vi "Main.vi"() -> ()   [LabVIEW 2019]
uses:
  Controls/Custom Calendar/Custom Calendar.xctl
  Controls/State Variables/Add User States.ctl
  Controls/State Variables/Edit User States.ctl
  Controls/State Variables/Add Item States.ctl
  Controls/State Variables/Edit Item States.ctl
  Controls/State Variables/Return Item States.ctl
  Controls/State Variables/Search Database States.ctl
  Controls/State Variables/User Item States.ctl
  Controls/State Variables/Main States.ctl
  Controls/State Variables/Edit Items States.ctl
  Controls/State Variables/Check Out Items States.ctl
  Controls/State Variables/Transfer Items States.ctl
  Controls/State Variables/Settings States.ctl
  Controls/State Variables/PSC Sales States.ctl
  Controls/References Cluster.ctl
  Controls/General Check Out Options.ctl
  <vilib>/event_ctls.llb/eventvkey.ctl
  <vilib>/vision/Image Controls.llb/IMAQ Image.ctl
  Controls/Table Data Types/Inventory Data Type.ctl
panel:
  in  "USER/ITEM DATA TRANSFER":T1(array[cluster])
  in  "PSC SALES MAIN STATE":T2
  in  "Settings State":T3
  in  "EMAILS SENT?":bool=TRUE
  in  "TRANSFER ITEMS STATE":T4
  in  "CHECK OUT ITEMS STATE":T5
  in  "EDIT ITEMS STATE":T6
  in  "Anticipate Graduation Year Map":map{string, i32}(c390)
  in  "Status Map":map{string, i32}(c390)
  in  "Department Map":map{string, i32}(c390)
  in  "Main State":T7
  in  "USER ITEMS STATE":T8
  in  "Search Database State":T9=enum."IDLE"
  out "Picture File Name":string
  out "BYU ID":string
  in  "RETURN ITEM STATE":T10
  in  "EDIT ITEM STATE":T11
  in  "ADD ITEM STATE":T12
  in  "EDIT USER STATE":T13
  in  "ADD USER STATE":T14
  in  "SEARCH DATABASE":bool
  in  "ADD ITEM":bool
  in  "ADD USER":bool
  in  "PSC SALES":bool
  in  "Main Pages":T15(tab)
  in  "Edit Database Settings":bool
  in  "RETURN ITEM":string
  in  "CLOSE":bool
  in  "DOWNLOAD USER PHOTO":bool
  in  "TAKE PHOTO USER":bool
  in  "User Comments":string
  in  "User Agreement":bool
  in  "CANCEL USER":bool
  in  "SAVE AND CLOSE USER":bool
  out "Add/Edit User Image":T16(plugin-control)
  out "Credit Score":string
  out "Graduation Clearance Date":string
  out "Date Added":string
  in  "Anticipated Graduation Year (Click to Select)":u16(ring) items=["2021", "2022", "2023", "2024", "2025", "2026", "2027", "2028", "2029", "2030"]
  in  "Status (Click to Select)":u16(ring) items=["Undergraduate", "Graduate", "Faculty/Staff"]
  in  "Department (Click to Select)":u16(ring) items=["ME", "EE", "CE", "CHEME", "MFGEN", "Other"]
  in  "Email (which you actually check)":string
  in  "Phone (###-###-####)":string
  in  "Last Name":string
  in  "First Name":string
  in  "BYU ID # (##-###-####)":string
  out "ADD/EDIT USER LABEL":string="ADD USER"
  in  "Camera":refnum<k21>
  in  "Reminder Notes":string
  in  "Archive Item Inputs":T17 {"Disposal Method" items=["Auction", "Sale", "Surplus", "Trash", "Other"]}
  in  "ARCHIVE ITEM":bool
  in  "CANCEL ITEM":bool
  in  "SAVE AND CLOSE ITEM":bool
  out "Most Recent Reminder Date":string
  out "Reminder Count":string
  out "Check Out Location":string
  out "Due Date":string
  out "Checked Out Date":string
  in  "Comments":string
  in  "Date Acquired":string
  in  "Serial #":string
  in  "Model #":string
  in  "Manufacturer":string
  in  "Manual":string
  in  "Location":string
  in  "Room":string
  in  "Item Description":string
  in  "BYU ICN #":string
  in  "ME #":string
  out "ADD/EDIT ITEM LABEL":string="ADD ITEM"
  in  "CANCEL RETURN ITEMS":bool
  in  "RETURN SELECTED ITEMS":bool
  in  "Item":string
  in  "What are you searching for?":u16(ring) items=["Identifier", "BYU ICN", "Item Description"]
  in  "Search Return Results":i32[](listbox)
  in  "Edit Sale Description":bool
  in  "Search Print Receipt":bool
  in  "Date Range":u16(ring) items=["Greater Than", "Less Than", "Between"]
  in  "Dates Less Than":string(xcontrol)
  in  "Dates Greater Than":string(xcontrol)
  in  "RESTORE USER":bool
  in  "CLOSE SEARCH":bool
  in  "EXPORT TO CLIPBOARD":bool
  in  "OPEN ITEM":bool
  in  "Sales Tracking Column Selector":T18={"SALE ID #"=TRUE, "BYU ID CARD #"=TRUE, "Sale Description"=TRUE, "Grand Total"=TRUE, "SALE DATE"=TRUE, "ITEM DESCRIPTION"=TRUE, "ITEM UNIT PRICE"=TRUE, "ITEM TOTAL PRICE"=TRUE, "ITEM QUANTITY"=TRUE, "SALE SEMESTER"=TRUE}
  in  "User Archive Column Selector":T19={"BYU ID #"=TRUE, "FIRST NAME"=TRUE, "LAST NAME"=TRUE, "PHONE NUMBER"=FALSE, "EMAIL"=FALSE, "DEPARTMENT"=TRUE, "STATUS"=TRUE, "ANTICIPATED GRADUATION YEAR"=TRUE, "CREDIT SCORE"=FALSE, "DATE ADDED"=TRUE, "GRADUATION CLEARANCE DATE"=TRUE, "USER PROFILE PICTURE PATH"=FALSE, "DATE ARCHIVED"=TRUE}
  in  "Inventory Archive Column Selector":T20={"DATE DISPOSED"=TRUE, "DISPOSAL METHOD"=TRUE, "AUCTION #"=TRUE, "DATE INVENTORY OFFICE EMAILED"=TRUE, "DISPOSAL NOTES"=TRUE, "IDENTIFIER"=TRUE, "BYU ICN #"=TRUE, "ITEM"=TRUE, "COMMENTS"=TRUE, "BUILDING/ROOM"=FALSE, "LOCATION IN ROOM"=FALSE, "MANUAL"=FALSE, "MANUFACTURER"=FALSE, "MODEL #"=FALSE, "SERIAL #"=FALSE, "DATE ACQUIRED"=TRUE}
  in  "User Column Selector":T21={"BYU ID #"=TRUE, "FIRST NAME"=TRUE, "LAST NAME"=TRUE, "PHONE NUMBER"=TRUE, "EMAIL"=TRUE, "DEPARTMENT"=TRUE, "GRADUATION STATUS"=TRUE, "ANTICIPATED GRADUATION YEAR"=FALSE, "CREDIT SCORE"=TRUE, "DATE ADDED"=FALSE, "GRADUATION CLEARANCE DATE"=FALSE, "PICTURE FILE NAME"=FALSE, "PICTURE FILE NAME 2"=FALSE}
  in  "Inventory Column Selector":T22={"IDENTIFIER"=TRUE, "BYU ICN #"=TRUE, "ITEM"=TRUE, "BUILDING/ROOM"=FALSE, "LOCATION IN ROOM"=FALSE, "MANUAL"=TRUE, "MANUFACTURER"=FALSE, "MODEL #"=FALSE, "SERIAL #"=FALSE, "DATE ACQUIRED"=FALSE, "BYU ID"=TRUE, "FIRST NAME"=TRUE, "LAST NAME"=TRUE, "CHECK OUT LOCATION"=TRUE, "CHECKED OUT DATE"=TRUE, "DUE DATE"=TRUE, "REMINDER COUNT"=TRUE, "MOST RECENT REMINDER DATE"=TRUE, "COMMENTS"=FALSE, "REMINDER NOTES"=FALSE}
  in  "COLUMNS TO VIEW":bool
  in  "OPEN USER":bool
  in  "Search Database Results":i32(listbox)
  in  "Column to Sort By":u16(ring) items=["BYU ID #", "First Name", "Last Name", "Phone Number", "Email", "Department", "Graduation Status", "Anticipated Graduation Year", "Credit Score", "Date Added", "Graduation Clearance Date", "User Profile Picture Path"]
  in  "Column to Search In":u16(ring) items=["BYU ID #", "First Name", "Last Name", "Phone Number", "Email", "Department", "Graduation Status", "Anticipated Graduation Year", "Credit Score", "Date Added", "Graduation Clearance Date", "User Profile Picture Path"]
  in  "What to Search For:":string
  in  "Where to Search":u16(ring) items=["Inventory", "Users", "Checked Out Items", "Inventory Archive", "User Archive", "Checked In Archive", "Sales Tracking", "Sales Archive"]
  in  "Checked In Archive Selector":T23={"ME #/ID #"=TRUE, "BYU ICN #"=TRUE, "ITEM DESCRIPTION"=TRUE, "BUILDING/ROOM"=FALSE, "LOCATION IN ROOM"=FALSE, "MANUAL"=TRUE, "MANUFACTURER"=FALSE, "MODEL #"=FALSE, "SERIAL #"=FALSE, "DATE ACQUIRED"=FALSE, "BYU ID #"=TRUE, "FIRST NAME"=TRUE, "LAST NAME"=TRUE, "CHECK OUT LOCATION"=TRUE, "CHECKED OUT DATE"=TRUE, "DUE DATE"=TRUE, "DATE RETURNED"=TRUE, "REMINDER COUNT"=FALSE, "MOST RECENT REMINDER DATE"=FALSE, "COMMENTS"=FALSE, "REMINDER NOTES"=FALSE}
  in  "SEE USER INFO COMMENTS":bool
  in  "User Info Comments":string
  in  "CHECK OUT ITEMS":bool
  in  "LOG OUT USER":bool
  in  "ARCHIVE USER":bool
  in  "EDIT USER":bool
  in  "EDIT SELECTED ITEMS":bool
  in  "TRANSFER SELECTED ITEMS":bool
  in  "USER RETURN SELECTED ITEMS":bool
  in  "User's Checked Out Items":i32[](listbox)
  in  "USER'S INFO":T24
  in  "USER EXPORT TO CLIPBOARD":bool
  in  "Altered Item Description":string
  in  "Possible Items":i32(listbox)
  in  "FINISH CHECK OUT ITEMS":bool
  in  "REMOVE SELECTED ITEMS":bool
  in  "CANCEL CHECK OUT ITEMS":bool
  in  "Items to be Checked Out":i32[](listbox)
  in  "Enter Item:":string
  in  "Check Out Location Selection":string
  in  "CHECK OUT STATICS":bool
  in  "CHECK OUT TODAY":bool
  in  "CHECK OUT END OF SEMESTER":bool
  in  "CHECK OUT MEASUREMENTS":bool
  in  "CHECK OUT MECHATRONICS":bool
  in  "Check Out Items Due Date":string(xcontrol)
  in  "New Item Description":string
  in  "New Reminder Notes":string
  in  "EDIT ITEMS SAVE AND CLOSE":bool
  in  "Items to Edit":i32[](listbox)
  in  "CANCEL EDIT ITEMS":bool
  in  "EDIT ITEMS REMOVE SELECTED ITEMS":bool
  in  "New Check Out Location":string
  in  "Edit Items Due Date":string(xcontrol)
  in  "EDIT ITEMS END OF SEMESTER":bool
  in  "EDIT ITEMS MECHATRONICS":bool
  in  "EDIT ITEMS STATICS":bool
  in  "EDIT ITEMS MEASUREMENTS":bool
  in  "TODAY EDIT ITEMS":bool
  in  "TRANSFER ITEMS":bool
  in  "Matching Individuals":i32(listbox)
  in  "TRANSFER ITEM REMOVE SELECTED ITEMS":bool
  in  "CANCEL TRANSFER ITEMS":bool
  in  "Items to be Transferred":i32[](listbox)
  in  "What to Match":u16(ring) items=["Last Name", "First Name", "BYU ID #"]
  in  "Search Parameter":string
  in  "Print Receipt":bool
  in  "CUSTOM ITEM":bool
  in  "Item List":i32[](listbox)
  in  "SAVE SALE AND CLOSE":bool
  out "Grand Total":string
  in  "BYU ID CARD #":string
  in  "Sale Description":string
  in  "Items to be Sold":i32[](listbox)
  in  "CANCEL ITEM SALE":bool
  in  "REMOVE SELECTED ITEMS SALES":bool
  in  "RUN CHARGE":bool
  in  "Scan or Enter Item Name":string
  in  "REMOVE SALE ITEM":bool
  in  "ADD NEW SALES ITEM":bool
  in  "PSC Sales Item Spreadsheet":string[][](table)
  in  "CANCEL EDIT SETTINGS":bool
  in  "Update Settings":bool
  in  "PSC Database Settings":string[][](table)
  in  "Enable or Disable Emails \n(Make sure only one computer has this enabled)":enum16{"ENABLE EMAILS", "DISABLE EMAILS"}(ring)
  # "Project Support Center\nDatabase Version 5.1.11"
  # "By checking this box I agree to return items in a prompt manner \nand will pay any late fees or replacement costs for late, broken or non-returned items.\nI also acknowledge that failure to return items could inhibit my ability to register for \nclasses and graduate - 12/5/2023"
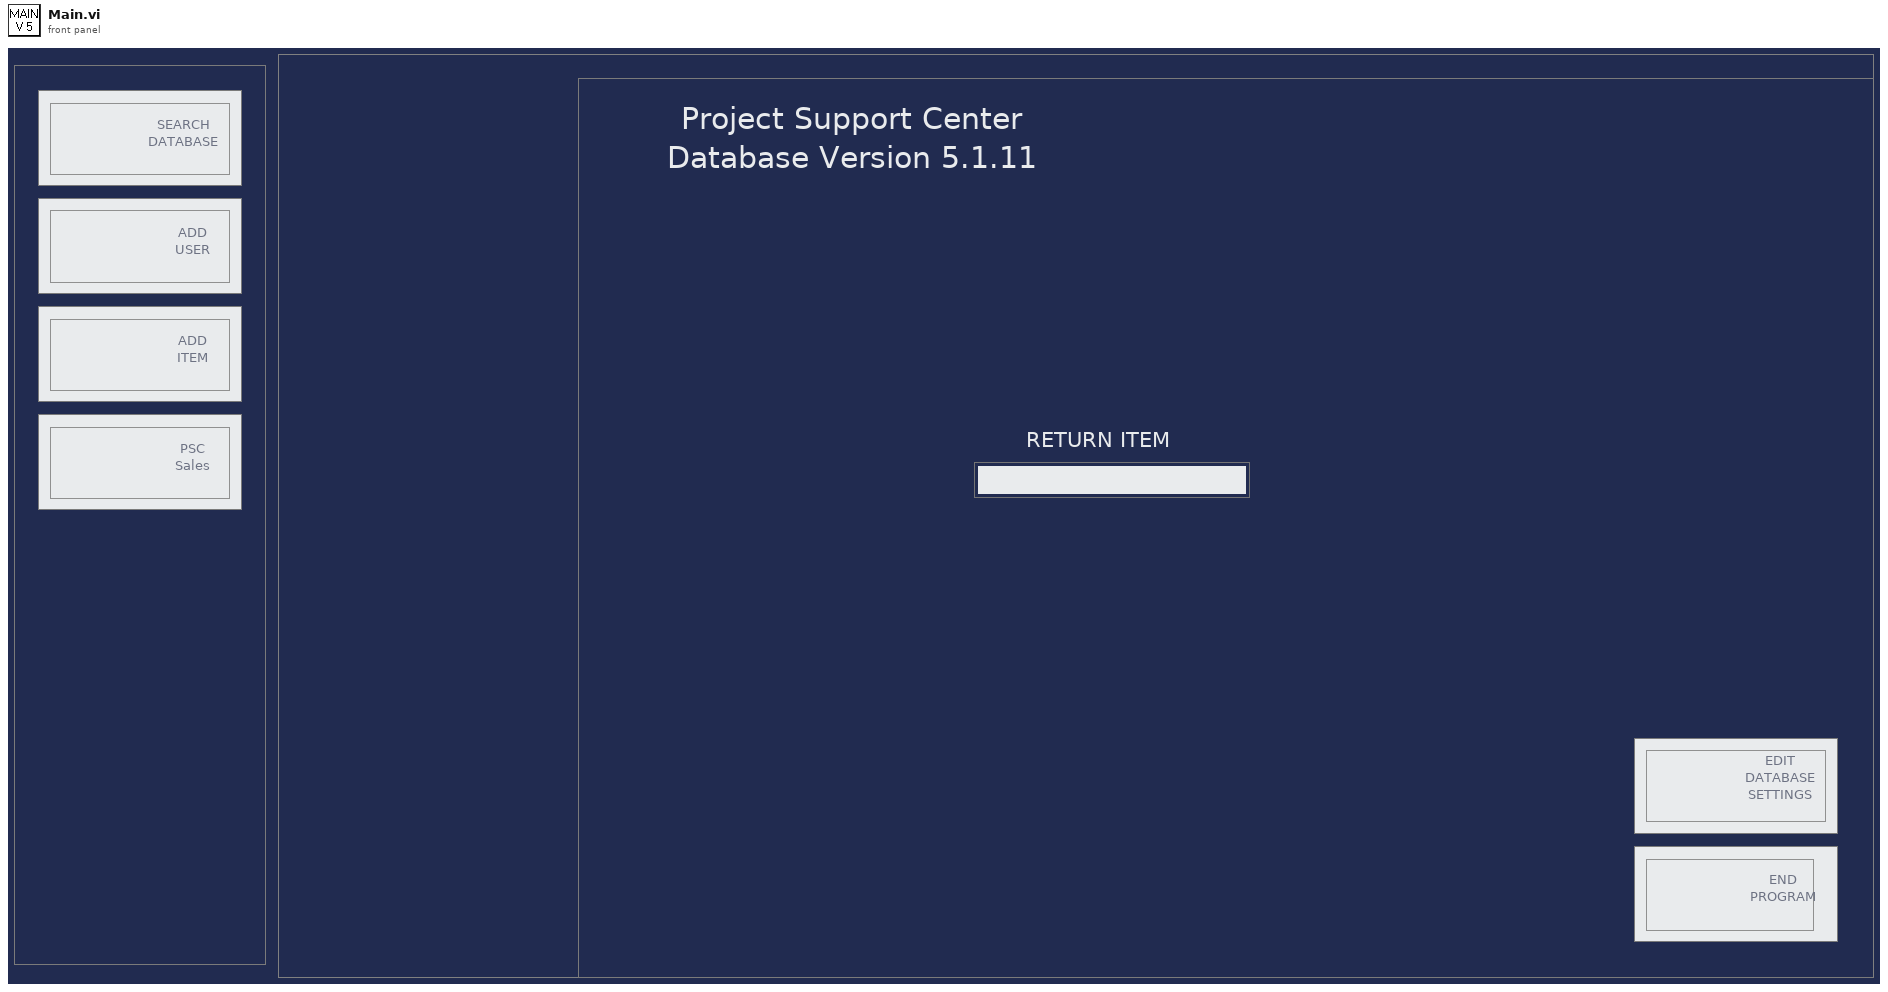
[diagram p1: front panel]
types:
  T1 = cluster{"DATA TYPE":enum16{"BYU ID", "ME#/IDENTIFIER", "BYU ICN"}, "DATA":string}[]
  T2 = typedef "PSC Sales States.ctl" = enum16{"INIT", "IDLE", "SEARCH ITEM LIST", "CUSTOM ITEM", "GET QUANTITY", "REMOVE ITEMS", "RUN CHARGE", "PRINT RECEIPT", "SAVE SALE", "END"}
  T3 = typedef "Settings States.ctl" = enum16{"INIT", "IDLE", "ADD SALE ITEM", "REMOVE SALE ITEM", "UPDATE SETTINGS", "END"}
  T4 = typedef "Transfer Items States.ctl" = enum16{"INIT", "IDLE", "FIND USER", "CONFIRM SELECTION", "REMOVE ITEMS", "TRANSFER ITEMS", "END"}
  T5 = typedef "Check Out Items States.ctl" = enum16{"INIT", "IDLE", "UPDATE SEARCH", "ADD ITEM", "EDIT DUE DATE", "EDIT LOCATION", "REMOVE ITEMS", "EDIT ITEM DESCRIPTION", "CHECK OUT ITEMS", "END"}
  T6 = typedef "Edit Items States.ctl" = enum16{"INIT", "IDLE", "EDIT DUE DATE", "EDIT LOCATION", "EDIT NOTES", "EDIT ITEM DESCRIPTION", "REMOVE ITEMS", "EDIT ITEMS", "END"}
  T7 = typedef "Main States.ctl" = enum16{"INIT", "IDLE", "ADD USER", "EDIT USER", "ADD ITEM", "EDIT ITEM", "RETURN ITEMS", "SEARCH DATABASE", "USER ITEMS", "EDIT ITEMS", "CHECK OUT ITEMS", "TRANSFER ITEMS", "PSC SALES", "ATRIUM", "INVENTORY TRACKING", "SETTINGS", "REMINDER EMAILS", "END"}
  T8 = typedef "User Item States.ctl" = enum16{"INIT", "IDLE", "GET USER ITEMS", "EDIT SELECTED ITEMS", "RETURN SELECTED ITEMS", "TRANSFER SELECTED ITEMS", "EDIT ALL ITEMS", "RETURN ALL ITEMS", "TRANSFER ALL ITEMS", "CHECK OUT ITEMS", "EDIT USER", "ARCHIVE USER", "END"}
  T9 = typedef "Search Database States.ctl" = enum16{"INIT", "IDLE", "UPDATE COLUMNS", "SEARCH DATABASE", "OPEN USER", "OPEN ITEM", "RESTORE USER", "PRINT SALE RECEIPT", "EDIT SALE DESCRIPTION", "END"}
  T10 = typedef "Return Item States.ctl" = enum16{"INIT", "IDLE", "SEARCH ITEMS", "RETURN ITEMS", "END"}
  T11 = typedef "Edit Item States.ctl" = enum16{"INIT", "IDLE", "EDIT ITEM", "ARCHIVE ITEM", "END"}
  T12 = typedef "Add Item States.ctl" = enum16{"INIT", "IDLE", "ADD ITEM", "END"}
  T13 = typedef "Edit User States.ctl" = enum16{"INIT", "IDLE", "TAKE PHOTO", "GET PHOTO", "EDIT USER", "END"}
  T14 = typedef "Add User States.ctl" = enum16{"INIT", "IDLE", "TAKE PHOTO", "GET PHOTO", "ADD USER", "END"}
  T15 = enum32{"IDLE", "ADD/EDIT USER", "ADD/EDIT ITEM", "RETURN ITEMS", "SEARCH DATABASE", "USER ITEMS", "CHECK OUT ITEMS", "EDIT ITEMS", "TRANSFER ITEMS", "PSC SALES", "ATRIUM", "INVENTORY TRACKING", "SETTINGS"}
  T16 = typedef "IMAQ Image.ctl" = refnum<image>
  T17 = cluster{"Disposal Date":string, "Disposal Method":u16, "Auction # / Other":string, "Date Disposal Email Sent":string, "Disposal Notes":string}
  T18 = cluster{"SALE ID #":bool, "BYU ID CARD #":bool, "Sale Description":bool, "Grand Total":bool, "SALE DATE":bool, "ITEM DESCRIPTION":bool, "ITEM UNIT PRICE":bool, "ITEM TOTAL PRICE":bool, "ITEM QUANTITY":bool, "SALE SEMESTER":bool}
  T19 = cluster{"BYU ID #":bool, "FIRST NAME":bool, "LAST NAME":bool, "PHONE NUMBER":bool, "EMAIL":bool, "DEPARTMENT":bool, "STATUS":bool, "ANTICIPATED GRADUATION YEAR":bool, "CREDIT SCORE":bool, "DATE ADDED":bool, "GRADUATION CLEARANCE DATE":bool, "USER PROFILE PICTURE PATH":bool, "DATE ARCHIVED":bool}
  T20 = cluster{"DATE DISPOSED":bool, "DISPOSAL METHOD":bool, "AUCTION #":bool, "DATE INVENTORY OFFICE EMAILED":bool, "DISPOSAL NOTES":bool, "IDENTIFIER":bool, "BYU ICN #":bool, "ITEM":bool, "COMMENTS":bool, "BUILDING/ROOM":bool, "LOCATION IN ROOM":bool, "MANUAL":bool, "MANUFACTURER":bool, "MODEL #":bool, "SERIAL #":bool, "DATE ACQUIRED":bool}
  T21 = cluster{"BYU ID #":bool, "FIRST NAME":bool, "LAST NAME":bool, "PHONE NUMBER":bool, "EMAIL":bool, "DEPARTMENT":bool, "GRADUATION STATUS":bool, "ANTICIPATED GRADUATION YEAR":bool, "CREDIT SCORE":bool, "DATE ADDED":bool, "GRADUATION CLEARANCE DATE":bool, "PICTURE FILE NAME":bool, "PICTURE FILE NAME 2":bool}
  T22 = cluster{"IDENTIFIER":bool, "BYU ICN #":bool, "ITEM":bool, "BUILDING/ROOM":bool, "LOCATION IN ROOM":bool, "MANUAL":bool, "MANUFACTURER":bool, "MODEL #":bool, "SERIAL #":bool, "DATE ACQUIRED":bool, "BYU ID":bool, "FIRST NAME":bool, "LAST NAME":bool, "CHECK OUT LOCATION":bool, "CHECKED OUT DATE":bool, "DUE DATE":bool, "REMINDER COUNT":bool, "MOST RECENT REMINDER DATE":bool, "COMMENTS":bool, "REMINDER NOTES":bool}
  T23 = cluster{"ME #/ID #":bool, "BYU ICN #":bool, "ITEM DESCRIPTION":bool, "BUILDING/ROOM":bool, "LOCATION IN ROOM":bool, "MANUAL":bool, "MANUFACTURER":bool, "MODEL #":bool, "SERIAL #":bool, "DATE ACQUIRED":bool, "BYU ID #":bool, "FIRST NAME":bool, "LAST NAME":bool, "CHECK OUT LOCATION":bool, "CHECKED OUT DATE":bool, "DUE DATE":bool, "DATE RETURNED":bool, "REMINDER COUNT":bool, "MOST RECENT REMINDER DATE":bool, "COMMENTS":bool, "REMINDER NOTES":bool}
  T24 = cluster{"BYU ID #":string, "First Name":string, "Last Name":string, "Phone Number":string, "Email":string, "Department":string, "Graduation Status":string, "Grad Year":string, "Credit Score":string, "Date Added":string, "Graduation Clearance Date":string, "User Items Photo":T16}
  T25 = typedef "References Cluster.ctl" = cluster{"MAIN PAGES":refnum<vi>, "ADD/EDIT ITEM REFERENCES":cluster{"Identifier":refnum<vi>, "BYU ICN #":refnum<vi>, "Item Description":refnum<vi>, "Comments":refnum<vi>, "Checked Out Date":refnum<vi>, "Due Date":refnum<vi>, "Check Out Location":refnum<vi>, "Reminder Count":refnum<vi>, "Most Recent Reminder Date":refnum<vi>, "BYU ID #":refnum<vi>, "Building/Room":refnum<vi>, "Location in Room":refnum<vi>, "Manual":refnum<vi>, "Manufacturer":refnum<vi>, "Model #":refnum<vi>, "Serial #":refnum<vi>, "Date Acquired":refnum<vi>, "ADD/EDIT ITEM LABEL":refnum<vi>, "ARCHIVE ITEM":refnum<vi>, "Archive Item Inputs":refnum<vi>, "Reminder Notes":refnum<vi>}, "ADD/EDIT USER REFERENCES":cluster{"BYU ID # (##-###-####)":refnum<vi>, "First Name":refnum<vi>, "Last Name":refnum<vi>, "Phone Number (###-###-####)":refnum<vi>, "Email":refnum<vi>, "Department":refnum<vi>, "Graduation Status":refnum<vi>, "Anticipated Graduation Year":refnum<vi>, "Credit Score":refnum<vi>, "Date Added":refnum<vi>, "Graduation Clearance Date":refnum<vi>, "Picture File Name":refnum<vi>, "ADD/EDIT USER LABEL":refnum<vi>, "Department Map":refnum<vi>, "Status Map":refnum<vi>, "Anticipated Graduation Year Map":refnum<vi>, "User Agreement":refnum<vi>, "User Comments":refnum<vi>, "Camera":refnum<vi>}, "RETURN ITEM REFERENCES":cluster{"Item or Person:":refnum<vi>, "Search Return Results":refnum<vi>, "What are you searching for?":refnum<vi>}, "SEARCH DATABASE REFERENCES":cluster{"What to Search For:":refnum<vi>, "Where to Search":refnum<vi>, "Column to Search In":refnum<vi>, "Column to Sort By":refnum<vi>, "Search Database Results":refnum<vi>, "Inventory Column Selector":refnum<vi>, "User Column Selector":refnum<vi>, "Inventory Archive Column Selector":refnum<vi>, "User Archive Column Selector":refnum<vi>, "Sales Tracking Column Selector":refnum<vi>, "Checked In Archive Column Selector":refnum<vi>, "Restore User":refnum<vi>, "Date Range":refnum<vi>, "Dates Less Than":refnum<vi>, "Dates Greater Than":refnum<vi>, "Search Print Receipt":refnum<vi>, "Edit Sale Description":refnum<vi>}, "USER ITEMS REFERENCES":cluster{"USER'S INFORMATION":refnum<vi>, "User's Checked Out Items":refnum<vi>, "User Info Comments":refnum<vi>, "SEE USER INFO COMMENTS":refnum<vi>}, "EDIT ITEMS REFERENCES":cluster{"New Check Out Location":refnum<vi>, "Items to Edit":refnum<vi>, "Edit Items Due Date":refnum<vi>, "New Reminder Notes":refnum<vi>, "New Item Description":refnum<vi>}, "CHECK OUT ITEMS REFERENCES":cluster{"Enter Item:":refnum<vi>, "Check Out Items Due Date":refnum<vi>, "Check Out Location":refnum<vi>, "Items to be Checked Out":refnum<vi>, "Possible Items":refnum<vi>, "Altered Item Description":refnum<vi>}, "TRANSFER ITEMS REFERENCES":cluster{"Search Parameter":refnum<vi>, "What to Match":refnum<vi>, "Matching Individuals":refnum<vi>, "Items to be Transferred":refnum<vi>}, "SETTINGS REFERENCES":cluster{"PSC Database Settings":refnum<vi>, "PSC Sales Item Spreadsheet":refnum<vi>}, "PSC SALES REFERENCES":cluster{"BYU ID CARD #":refnum<vi>, "Sale Description":refnum<vi>, "Scan or Enter Item Name":refnum<vi>, "Items to be Sold":refnum<vi>, "Grand Total":refnum<vi>, "Item List":refnum<vi>}}
  T26 = cluster{"Identifier":refnum<vi>, "BYU ICN #":refnum<vi>, "Item Description":refnum<vi>, "Comments":refnum<vi>, "Checked Out Date":refnum<vi>, "Due Date":refnum<vi>, "Check Out Location":refnum<vi>, "Reminder Count":refnum<vi>, "Most Recent Reminder Date":refnum<vi>, "BYU ID #":refnum<vi>, "Building/Room":refnum<vi>, "Location in Room":refnum<vi>, "Manual":refnum<vi>, "Manufacturer":refnum<vi>, "Model #":refnum<vi>, "Serial #":refnum<vi>, "Date Acquired":refnum<vi>, "ADD/EDIT ITEM LABEL":refnum<vi>, "ARCHIVE ITEM":refnum<vi>, "Archive Item Inputs":refnum<vi>, "Reminder Notes":refnum<vi>}
  T27 = cluster{"BYU ID # (##-###-####)":refnum<vi>, "First Name":refnum<vi>, "Last Name":refnum<vi>, "Phone Number (###-###-####)":refnum<vi>, "Email":refnum<vi>, "Department":refnum<vi>, "Graduation Status":refnum<vi>, "Anticipated Graduation Year":refnum<vi>, "Credit Score":refnum<vi>, "Date Added":refnum<vi>, "Graduation Clearance Date":refnum<vi>, "Picture File Name":refnum<vi>, "ADD/EDIT USER LABEL":refnum<vi>, "Department Map":refnum<vi>, "Status Map":refnum<vi>, "Anticipated Graduation Year Map":refnum<vi>, "User Agreement":refnum<vi>, "User Comments":refnum<vi>, "Camera":refnum<vi>}
  T28 = cluster{"Item or Person:":refnum<vi>, "Search Return Results":refnum<vi>, "What are you searching for?":refnum<vi>}
  T29 = cluster{"What to Search For:":refnum<vi>, "Where to Search":refnum<vi>, "Column to Search In":refnum<vi>, "Column to Sort By":refnum<vi>, "Search Database Results":refnum<vi>, "Inventory Column Selector":refnum<vi>, "User Column Selector":refnum<vi>, "Inventory Archive Column Selector":refnum<vi>, "User Archive Column Selector":refnum<vi>, "Sales Tracking Column Selector":refnum<vi>, "Check In Archive Column Selector":refnum<vi>, "Restore User":refnum<vi>, "Date Range":refnum<vi>, "Dates Less Than":refnum<vi>, "Dates Greater Than":refnum<vi>, "Search Print Receipt":refnum<vi>, "Edit Sale Description":refnum<vi>}
  T30 = cluster{"USER'S INFORMATION":refnum<vi>, "User's Checked Out Items":refnum<vi>, "User Info Comments":refnum<vi>, "SEE USER INFO COMMENTS":refnum<vi>}
  T31 = cluster{"New Check Out Location":refnum<vi>, "Items to Edit":refnum<vi>, "Edit Items Due Date":refnum<vi>, "New Reminder Notes":refnum<vi>, "New Item Description":refnum<vi>}
  T32 = cluster{"Enter Item:":refnum<vi>, "Check Out Items Due Date":refnum<vi>, "Check Out Location":refnum<vi>, "Items to be Checked Out":refnum<vi>, "Possible Items":refnum<vi>, "Altered Item Description":refnum<vi>}
  T33 = cluster{"Search Parameter":refnum<vi>, "What to Match":refnum<vi>, "Matching Individuals":refnum<vi>, "Items to be Transferred":refnum<vi>}
  T34 = cluster{"PSC Database Settings":refnum<vi>, "PSC Sales Spreadsheet":refnum<vi>}
  T35 = cluster{"BYU ID CARD #":refnum<vi>, "Sale Description":refnum<vi>, "Scan Barcode":refnum<vi>, "Items to be Sold":refnum<vi>, "Grand Total":refnum<vi>, "Item List":refnum<vi>}
  T36 = cluster{"BYU ID #":string, "First Name":string, "Last Name":string, "Phone Number":string, "Email":string, "Department":u16, "Graduation Status":u16, "Anticipated Graduation Year":u16, "Credit Score":string, "Date Added":string, "Graduation Clearance Date":string, "Picture File Name":string, "User Comments":string}
  T37 = cluster{"Identifier":string, "BYU ICN #":string, "Item Description":string, "Comments":string, "Checked Out Date":string, "Due Date":string, "Check Out Location":string, "Reminder Count":string, "Most Recent Reminder Date":string, "BYU ID #":string, "Building/Room":string, "Location in Room":string, "Manual":string, "Manufacturer":string, "Model #":string, "Serial #":string, "Date Acquired":string, "Reminder Notes":string}
  T38 = typedef "Inventory Data Type.ctl" = cluster{"Identifier":string, "BYU ICN #":string, "Item Description":string, "Comments":string, "Checked Out Date":string, "Due Date":string, "Check Out Location":string, "Reminder Count":i32, "Most Recent Reminder Date":string, "BYU ID #":string, "Building/Room":string, "Location in Room":string, "Manual":string, "Manufacturer":string, "Model #":string, "Serial #":string, "Date Acquired":string, "Reminder Notes":string}
  T39 = cluster{"DATA TYPE":enum16{"BYU ID", "ME#/IDENTIFIER", "BYU ICN"}, "DATA":string}
  T40 = enum8{"Enabled", "Disabled", "Disabled and Grayed Out"}
  T41 = typedef "General Check Out Options.ctl" = enum16{"TODAY", "END OF SEMESTER", "MEASUREMENTS", "MECHATRONICS", "STATICS"}
  T42 = typedef "eventvkey.ctl" = enum16{"ASCII", "Enter", "Return", "Shift", "Ctrl", "Alt", "Cmd", "Opt", "Caps", "NumLock", "Clear", "Break", "Up", "Down", "Left", "Right", "Insert", "Delete", "Home", "End", "PageUp", "PageDown", "Escape", "Help", "Pause", "ScrollLock", "F1", "F2", "F3", "F4", "F5", "F6", "F7", "F8", "F9", "F10", "F11", "F12", "F13", "F14", "F15", "F16", "F17", "F18", "F19", "F20", "F21", "F22", "F23", "F24", "Play", "VolumeUp", "VolumeDown", "Mute", "Two Byte Char"}
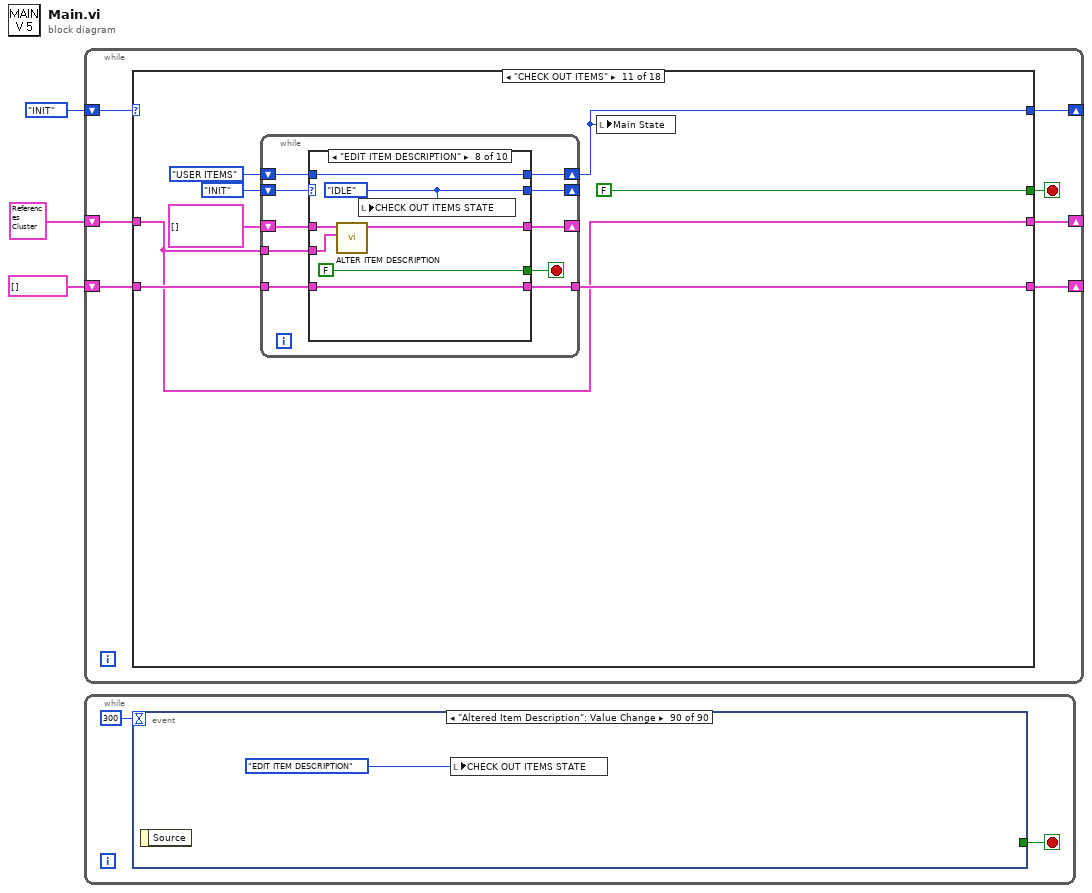
[diagram p0: block diagram]
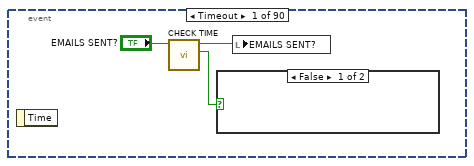
[diagram p2: hidden frame]
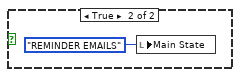
[diagram p3: hidden frame]
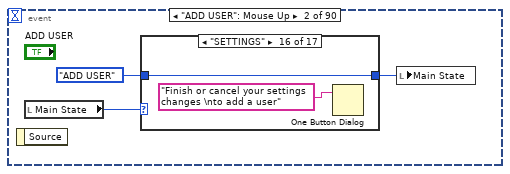
[diagram p4: hidden frame]
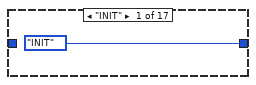
[diagram p5: hidden frame]
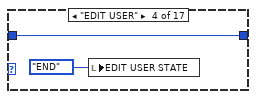
[diagram p8: hidden frame]
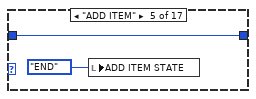
[diagram p9: hidden frame]
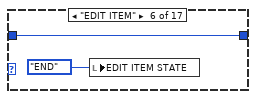
[diagram p10: hidden frame]
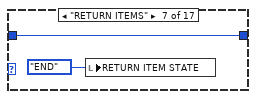
[diagram p11: hidden frame]
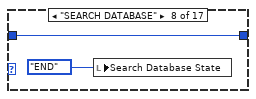
[diagram p12: hidden frame]
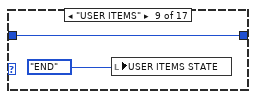
[diagram p13: hidden frame]
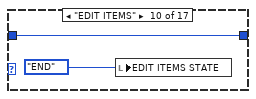
[diagram p14: hidden frame]
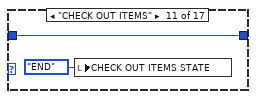
[diagram p15: hidden frame]
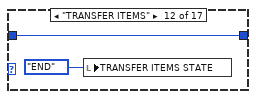
[diagram p16: hidden frame]
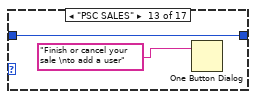
[diagram p17: hidden frame]
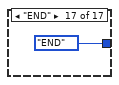
[diagram p20: hidden frame]
diagram:
  n1 = while {
    shift-right: [w6] -> _
    shift-left: Main_States."INIT" -> [w4]
    shift-right: [w8] -> _
    shift-left: T25 {"MAIN PAGES"=refnum, "ADD/EDIT ITEM REFERENCES"={"Identifier"=refnum, "BYU ICN #"=refnum, "Item Description"=refnum, "Comments"=refnum, "Checked Out Date"=refnum, "Due Date"=refnum, "Check Out Location"=refnum, "Reminder Count"=refnum, "Most Recent Reminder Date"=refnum, "BYU ID #"=refnum, "Building/Room"=refnum, "Location in Room"=refnum, "Manual"=refnum, "Manufacturer"=refnum, "Model #"=refnum, "Serial #"=refnum, "Date Acquired"=refnum, "ADD/EDIT ITEM LABEL"=refnum, "ARCHIVE ITEM"=refnum, "Archive Item Inputs"=refnum, "Reminder Notes"=refnum}, "ADD/EDIT USER REFERENCES"={"BYU ID # (##-###-####)"=refnum, "First Name"=refnum, "Last Name"=refnum, "Phone Number (###-###-####)"=refnum, "Email"=refnum, "Department"=refnum, "Graduation Status"=refnum, "Anticipated Graduation Year"=refnum, "Credit Score"=refnum, "Date Added"=refnum, "Graduation Clearance Date"=refnum, "Picture File Name"=refnum, "ADD/EDIT USER LABEL"=refnum, "Department Map"=refnum, "Status Map"=refnum, "Anticipated Graduation Year Map"=refnum, "User Agreement"=refnum, "User Comments"=refnum, "Camera"=refnum}, "RETURN ITEM REFERENCES"={"Item or Person:"=refnum, "Search Return Results"=refnum, "What are you searching for?"=refnum}, "SEARCH DATABASE REFERENCES"={"What to Search For:"=refnum, "Where to Search"=refnum, "Column to Search In"=refnum, "Column to Sort By"=refnum, "Search Database Results"=refnum, "Inventory Column Selector"=refnum, "User Column Selector"=refnum, "Inventory Archive Column Selector"=refnum, "User Archive Column Selector"=refnum, "Sales Tracking Column Selector"=refnum, "Checked In Archive Column Selector"=refnum, "Restore User"=refnum, "Date Range"=refnum, "Dates Less Than"=refnum, "Dates Greater Than"=refnum, "Search Print Receipt"=refnum, "Edit Sale Description"=refnum}, "USER ITEMS REFERENCES"={"USER'S INFORMATION"=refnum, "User's Checked Out Items"=refnum, "User Info Comments"=refnum, "SEE USER INFO COMMENTS"=refnum}, "EDIT ITEMS REFERENCES"={"New Check Out Location"=refnum, "Items to Edit"=refnum, "Edit Items Due Date"=refnum, "New Reminder Notes"=refnum, "New Item Description"=refnum}, "CHECK OUT ITEMS REFERENCES"={"Enter Item:"=refnum, "Check Out Items Due Date"=refnum, "Check Out Location"=refnum, "Items to be Checked Out"=refnum, "Possible Items"=refnum, "Altered Item Description"=refnum}, "TRANSFER ITEMS REFERENCES"={"Search Parameter"=refnum, "What to Match"=refnum, "Matching Individuals"=refnum, "Items to be Transferred"=refnum}, "SETTINGS REFERENCES"={"PSC Database Settings"=refnum, "PSC Sales Item Spreadsheet"=refnum}, "PSC SALES REFERENCES"={"BYU ID CARD #"=refnum, "Sale Description"=refnum, "Scan or Enter Item Name"=refnum, "Items to be Sold"=refnum, "Grand Total"=refnum, "Item List"=refnum}} ("REFERENCES") -> [w9]
    shift-right: [w5] -> _
    shift-left: T1 [] ("USER/ITEM DATA TRANSFER") -> [w7]
    stop <- w10 stop-if-true
    n2 = case shown="\"CHECK OUT ITEMS\"" w4 {
      tunnel: [FALSE FALSE FALSE FALSE FALSE FALSE w420 FALSE FALSE FALSE FALSE FALSE FALSE FALSE FALSE FALSE FALSE TRUE] -> w10
      tunnel: w9 -> [w15 w166 w174 w263 w338 w376 w421 w450 w543 w658 w743 w840 w922 w965 w970 w976 w1014 w1018]
      tunnel: [w14 w166 w174 w263 w338 w376 w421 w450 w543 w658 w743 w840 w922 w965 w970 w973 w1014 w1018] -> w8
      tunnel: w7 -> [w12 _ w169 w261 w334 w374 w419 w452 w541 w652 w747 w843 w923 w964 w969 w975 w1015 _]
      tunnel: [w11 "Main State" w171 w258 w335 w372 w418 w446 w539 w654 w742 w836 w919 w963 w967 w971 w1012 Main_States."END"] -> w6
      tunnel: [w12 "USER/ITEM DATA TRANSFER" w168 w257 w334 w374 w419 w449 w538 w656 w745 w841 w923 w964 w969 w974 w1015 T1 [] ("USER/ITEM DATA TRANSFER")] -> w5
      frame "INIT", Default {
        w11 = Main_States."IDLE"
        n3 = for {
          N: 12 -> [_]
          shift-right: [w17] -> w14
          shift-left: w15 -> [w18]
          i -> [w19]
          n4 = case shown="7" w19 {
            tunnel: w18 -> [w27 w52 w62 w78 w103 w111 w119 w124 w132 w145 w151 w157]
            tunnel: [w25 w50 w68 w76 w91 w106 w117 w125 w133 w145 w150 w154] -> w17
            frame 0, Default {
              n5 = control-ref of="RETURN ITEM"() -> (w22:refnum<vi>)
              n6 = control-ref of="USER/ITEM DATA TRANSFER"() -> (w23:refnum<vi>)
              n7 = property class="Str"(reference=w22, "Value"="") -> ()  [unwired: 1 in, 2 out]
              n8 = local write "Main State"(Main_States."IDLE") -> ()
              n9 = property class="Arr (strict)"(reference=w23, "Value"=T1 []) -> ()  [unwired: 1 in, 2 out]
              n10 = control-ref of="Main Pages"() -> (w26:refnum<vi>)
              n11 = Bundle By Name(cluster=w27, "MAIN PAGES"=w26) -> (w25:T25)
            }
            frame 1 {
              n12 = control-ref of="ME #"() -> (w49:refnum<vi>)
              n13 = control-ref of="BYU ICN #"() -> (w48:refnum<vi>)
              n14 = control-ref of="Item Description"() -> (w47:refnum<vi>)
              n15 = control-ref of="Comments"() -> (w46:refnum<vi>)
              n16 = control-ref of="Checked Out Date"() -> (w45:refnum<vi>)
              n17 = control-ref of="Due Date"() -> (w44:refnum<vi>)
              n18 = control-ref of="Check Out Location"() -> (w43:refnum<vi>)
              n19 = control-ref of="Reminder Count"() -> (w42:refnum<vi>)
              n20 = control-ref of="Most Recent Reminder Date"() -> (w41:refnum<vi>)
              n21 = control-ref of="BYU ID #"() -> (w40:refnum<vi>)
              n22 = control-ref of="Building/Room"() -> (w39:refnum<vi>)
              n23 = control-ref of="Location in Room"() -> (w38:refnum<vi>)
              n24 = control-ref of="Manual"() -> (w37:refnum<vi>)
              n25 = control-ref of="Manufacturer"() -> (w36:refnum<vi>)
              n26 = control-ref of="Model #"() -> (w35:refnum<vi>)
              n27 = control-ref of="Serial #"() -> (w34:refnum<vi>)
              n28 = control-ref of="Date Acquired"() -> (w33:refnum<vi>)
              n29 = control-ref of="ADD/EDIT ITEM LABEL"() -> (w32:refnum<vi>)
              n30 = control-ref of="ARCHIVE ITEM"() -> (w31:refnum<vi>)
              n31 = control-ref of="Archive Item Inputs"() -> (w30:refnum<vi>)
              n32 = control-ref of="Reminder Notes"() -> (w28:refnum<vi>)
              n33 = Bundle(cluster=T26 {"Identifier"=refnum, "BYU ICN #"=refnum, "Item Description"=refnum, "Comments"=refnum, "Checked Out Date"=refnum, "Due Date"=refnum, "Check Out Location"=refnum, "Reminder Count"=refnum, "Most Recent Reminder Date"=refnum, "BYU ID #"=refnum, "Building/Room"=refnum, "Location in Room"=refnum, "Manual"=refnum, "Manufacturer"=refnum, "Model #"=refnum, "Serial #"=refnum, "Date Acquired"=refnum, "ADD/EDIT ITEM LABEL"=refnum, "ARCHIVE ITEM"=refnum, "Archive Item Inputs"=refnum, "Reminder Notes"=refnum} ("ADD/EDIT ITEM REFERENCES"), "Identifier"=w49, "BYU ICN #"=w48, "Item Description"=w47, "Comments"=w46, "Checked Out Date"=w45, "Due Date"=w44, "Check Out Location"=w43, "Reminder Count"=w42, "Most Recent Reminder Date"=w41, "BYU ID #"=w40, "Building/Room"=w39, "Location in Room"=w38, "Manual"=w37, "Manufacturer"=w36, "Model #"=w35, "Serial #"=w34, "Date Acquired"=w33, "ADD/EDIT ITEM LABEL"=w32, "ARCHIVE ITEM"=w31, "Archive Item Inputs"=w30, "Reminder Notes"=w28) -> (w51:T26)
              n34 = Bundle By Name(cluster=w52, "ADD/EDIT ITEM REFERENCES"=w51) -> (w50:T25)
            }
            frame 2 {
              n35 = control-ref of="Camera"() -> (w53:refnum<vi>)
              n36 = control-ref of="User Agreement"() -> (w56:refnum<vi>)
              n37 = control-ref of="BYU ID # (##-###-####)"() -> (w65:refnum<vi>)
              n38 = control-ref of="First Name"() -> (w75:refnum<vi>)
              n39 = control-ref of="Last Name"() -> (w74:refnum<vi>)
              n40 = control-ref of="Phone Number (###-###-####)"() -> (w73:refnum<vi>)
              n41 = control-ref of="Email (which you actually check)"() -> (w72:refnum<vi>)
              n42 = control-ref of="Credit Score"() -> (w61:refnum<vi>)
              n43 = control-ref of="Date Added"() -> (w60:refnum<vi>)
              n44 = control-ref of="Graduation Clearance Date"() -> (w59:refnum<vi>)
              n45 = control-ref of="Picture File Name"() -> (w58:refnum<vi>)
              n46 = control-ref of="ADD/EDIT USER LABEL"() -> (w57:refnum<vi>)
              n47 = control-ref of="User Comments"() -> (w55:refnum<vi>)
              n48 = control-ref of="Department (Click to Select)"() -> (w71:refnum<vi>)
              n49 = control-ref of="Graduation Status"() -> (w70:refnum<vi>)
              n50 = control-ref of="Anticipated Graduation Year (Click to Select)"() -> (w69:refnum<vi>)
              n51 = control-ref of="Department Map"() -> (w67:refnum<vi>)
              n52 = control-ref of="Status Map"() -> (w66:refnum<vi>)
              n53 = control-ref of="Anticipate Graduation Year Map"() -> (w64:refnum<vi>)
              n54 = Bundle(cluster=T27 {"BYU ID # (##-###-####)"=refnum, "First Name"=refnum, "Last Name"=refnum, "Phone Number (###-###-####)"=refnum, "Email"=refnum, "Department"=refnum, "Graduation Status"=refnum, "Anticipated Graduation Year"=refnum, "Credit Score"=refnum, "Date Added"=refnum, "Graduation Clearance Date"=refnum, "Picture File Name"=refnum, "ADD/EDIT USER LABEL"=refnum, "Department Map"=refnum, "Status Map"=refnum, "Anticipated Graduation Year Map"=refnum, "User Agreement"=refnum, "User Comments"=refnum, "Camera"=refnum} ("ADD/EDIT USER REFERENCES"), "BYU ID # (##-###-####)"=w65, "First Name"=w75, "Last Name"=w74, "Phone Number (###-###-####)"=w73, "Email"=w72, "Department"=w71, "Graduation Status"=w70, "Anticipated Graduation Year"=w69, "Credit Score"=w61, "Date Added"=w60, "Graduation Clearance Date"=w59, "Picture File Name"=w58, "ADD/EDIT USER LABEL"=w57, "Department Map"=w67, "Status Map"=w66, "Anticipated Graduation Year Map"=w64, "User Agreement"=w56, "User Comments"=w55, "Camera"=w53) -> (w63:T27)
              n55 = Bundle By Name(cluster=w62, "ADD/EDIT USER REFERENCES"=w63) -> (w68:T25)
            }
            frame 3 {
              n56 = control-ref of="Search Return Results"() -> (w80:refnum<vi>)
              n57 = control-ref of="Item"() -> (w81:refnum<vi>)
              n58 = control-ref of="What are you searching for?"() -> (w79:refnum<vi>)
              n59 = Bundle(cluster=T28 {"Item or Person:"=refnum, "Search Return Results"=refnum, "What are you searching for?"=refnum} ("RETURN ITEM REFERENCES"), "Item or Person:"=w81, "Search Return Results"=w80, "What are you searching for?"=w79) -> (w77:T28)
              n60 = Bundle By Name(cluster=w78, "RETURN ITEM REFERENCES"=w77) -> (w76:T25)
            }
            frame 4 {
              n61 = control-ref of="Search Database Results"() -> (w98:refnum<vi>)
              n62 = control-ref of="Dates Less Than"() -> (w87:refnum<vi>)
              n63 = control-ref of="Dates Greater Than"() -> (w86:refnum<vi>)
              n64 = control-ref of="Search Print Receipt"() -> (w85:refnum<vi>)
              n65 = control-ref of="Edit Sale Description"() -> (w83:refnum<vi>)
              n66 = control-ref of="Restore User"() -> (w89:refnum<vi>)
              n67 = control-ref of="Inventory Archive Column Selector"() -> (w95:refnum<vi>)
              n68 = control-ref of="Inventory Column Selector"() -> (w97:refnum<vi>)
              n69 = control-ref of="User Column Selector"() -> (w96:refnum<vi>)
              n70 = control-ref of="User Archive Column Selector"() -> (w94:refnum<vi>)
              n71 = control-ref of="Sales Tracking Column Selector"() -> (w93:refnum<vi>)
              n72 = control-ref of="Checked In Archive Selector"() -> (w90:refnum<vi>)
              n73 = control-ref of="What to Search For:"() -> (w102:refnum<vi>)
              n74 = control-ref of="Date Range"() -> (w88:refnum<vi>)
              n75 = control-ref of="Where to Search"() -> (w101:refnum<vi>)
              n76 = control-ref of="Column to Search In"() -> (w100:refnum<vi>)
              n77 = control-ref of="Column to Sort By"() -> (w99:refnum<vi>)
              n78 = Bundle(cluster=T29 {"What to Search For:"=refnum, "Where to Search"=refnum, "Column to Search In"=refnum, "Column to Sort By"=refnum, "Search Database Results"=refnum, "Inventory Column Selector"=refnum, "User Column Selector"=refnum, "Inventory Archive Column Selector"=refnum, "User Archive Column Selector"=refnum, "Sales Tracking Column Selector"=refnum, "Check In Archive Column Selector"=refnum, "Restore User"=refnum, "Date Range"=refnum, "Dates Less Than"=refnum, "Dates Greater Than"=refnum, "Search Print Receipt"=refnum, "Edit Sale Description"=refnum} ("SEARCH DATABASE REFERENCES"), "What to Search For:"=w102, "Where to Search"=w101, "Column to Search In"=w100, "Column to Sort By"=w99, "Search Database Results"=w98, "Inventory Column Selector"=w97, "User Column Selector"=w96, "Inventory Archive Column Selector"=w95, "User Archive Column Selector"=w94, "Sales Tracking Column Selector"=w93, "Check In Archive Column Selector"=w90, "Restore User"=w89, "Date Range"=w88, "Dates Less Than"=w87, "Dates Greater Than"=w86, "Search Print Receipt"=w85, "Edit Sale Description"=w83) -> (w92:T29)
              n79 = Bundle By Name(cluster=w103, "SEARCH DATABASE REFERENCES"=w92) -> (w91:T25)
            }
            frame 5 {
              n80 = control-ref of="User's Checked Out Items"() -> (w108:refnum<vi>)
              n81 = control-ref of="SEE USER INFO COMMENTS"() -> (w104:refnum<vi>)
              n82 = control-ref of="USER'S INFO"() -> (w109:refnum<vi>)
              n83 = control-ref of="User Info Comments"() -> (w105:refnum<vi>)
              n84 = Bundle(cluster=T30 {"USER'S INFORMATION"=refnum, "User's Checked Out Items"=refnum, "User Info Comments"=refnum, "SEE USER INFO COMMENTS"=refnum} ("USER ITEMS REFERENCES"), "USER'S INFORMATION"=w109, "User's Checked Out Items"=w108, "User Info Comments"=w105, "SEE USER INFO COMMENTS"=w104) -> (w107:T30)
              n85 = Bundle By Name(cluster=w111, "USER ITEMS REFERENCES"=w107) -> (w106:T25)
            }
            frame 6 {
              n86 = control-ref of="Items to Edit"() -> (w114:refnum<vi>)
              n87 = control-ref of="Edit Items Due Date"() -> (w115:refnum<vi>)
              n88 = control-ref of="New Check Out Location"() -> (w120:refnum<vi>)
              n89 = control-ref of="New Reminder Notes"() -> (w113:refnum<vi>)
              n90 = control-ref of="New Item Description"() -> (w112:refnum<vi>)
              n91 = Bundle(cluster=T31 {"New Check Out Location"=refnum, "Items to Edit"=refnum, "Edit Items Due Date"=refnum, "New Reminder Notes"=refnum, "New Item Description"=refnum} ("EDIT ITEMS REFERENCES"), "New Check Out Location"=w120, "Items to Edit"=w114, "Edit Items Due Date"=w115, "New Reminder Notes"=w113, "New Item Description"=w112) -> (w118:T31)
              n92 = Bundle By Name(cluster=w119, "EDIT ITEMS REFERENCES"=w118) -> (w117:T25)
            }
            frame 7 {
              n93 = control-ref of="Possible Items"() -> (w123:refnum<vi>)
              n94 = control-ref of="Items to be Checked Out"() -> (w127:refnum<vi>)
              n95 = control-ref of="Altered Item Description"() -> (w121:refnum<vi>)
              n96 = control-ref of="Check Out Items Due Date"() -> (w129:refnum<vi>)
              n97 = control-ref of="Enter Item:"() -> (w130:refnum<vi>)
              n98 = control-ref of="Check Out Location Selection"() -> (w128:refnum<vi>)
              n99 = Bundle(cluster=T32 {"Enter Item:"=refnum, "Check Out Items Due Date"=refnum, "Check Out Location"=refnum, "Items to be Checked Out"=refnum, "Possible Items"=refnum, "Altered Item Description"=refnum} ("CHECK OUT ITEMS REFERENCES"), "Enter Item:"=w130, "Check Out Items Due Date"=w129, "Check Out Location"=w128, "Items to be Checked Out"=w127, "Possible Items"=w123, "Altered Item Description"=w121) -> (w126:T32)
              n100 = Bundle By Name(cluster=w124, "CHECK OUT ITEMS REFERENCES"=w126) -> (w125:T25)
            }
            frame 8 {
              n101 = control-ref of="Matching Individuals"() -> (w136:refnum<vi>)
              n102 = control-ref of="Items to be Transferred"() -> (w135:refnum<vi>)
              n103 = control-ref of="Search Parameter"() -> (w138:refnum<vi>)
              n104 = control-ref of="What to Match"() -> (w137:refnum<vi>)
              n105 = Bundle(cluster=T33 {"Search Parameter"=refnum, "What to Match"=refnum, "Matching Individuals"=refnum, "Items to be Transferred"=refnum} ("TRANSFER ITEMS REFERENCES"), "Search Parameter"=w138, "What to Match"=w137, "Matching Individuals"=w136, "Items to be Transferred"=w135) -> (w134:T33)
              n106 = Bundle By Name(cluster=w132, "TRANSFER ITEMS REFERENCES"=w134) -> (w133:T25)
            }
            frame 9 {
              n107 = call "UPDATE MAPS.vi"("Anticipate Graduation Year Map In"="Anticipate Graduation Year Map", "Status Map In"="Status Map", "Department Map In"="Department Map", "REFERENCES"=w145) -> ("Anticipate Graduation Year Map Out"=w139:map{string, i32}, "Status Map Out"=w140:map{string, i32}, "Department Map Out"=w141:map{string, i32})  [unwired: 5 in]
              n108 = local write "Department Map"(w141) -> ()
              n109 = local write "Status Map"(w140) -> ()
              n110 = local write "Anticipate Graduation Year Map"(w139) -> ()
            }
            frame 10 {
              n111 = control-ref of="PSC Sales Item Spreadsheet"() -> (w146:refnum<vi>)
              n112 = control-ref of="PSC Database Settings"() -> (w149:refnum<vi>)
              n113 = Bundle(cluster=T34 {"PSC Database Settings"=refnum, "PSC Sales Spreadsheet"=refnum} ("output cluster"), "PSC Database Settings"=w149, "PSC Sales Spreadsheet"=w146) -> (w148:T34)
              n114 = Bundle By Name(cluster=w151, "SETTINGS REFERENCES"=w148) -> (w150:T25)
            }
            frame 11 {
              n115 = control-ref of="Grand Total"() -> (w153:refnum<vi>)
              n116 = control-ref of="Item List"() -> (w152:refnum<vi>)
              n117 = control-ref of="BYU ID CARD #"() -> (w161:refnum<vi>)
              n118 = control-ref of="Sale Description"() -> (w160:refnum<vi>)
              n119 = control-ref of="Scan or Enter Item Name"() -> (w159:refnum<vi>)
              n120 = control-ref of="Items to be Sold"() -> (w158:refnum<vi>)
              n121 = Bundle(cluster=T35 {"BYU ID CARD #"=refnum, "Sale Description"=refnum, "Scan Barcode"=refnum, "Items to be Sold"=refnum, "Grand Total"=refnum, "Item List"=refnum} ("PSC SALES REFERENCES"), "BYU ID CARD #"=w161, "Sale Description"=w160, "Scan Barcode"=w159, "Items to be Sold"=w158, "Grand Total"=w153, "Item List"=w152) -> (w156:T35)
              n122 = Bundle By Name(cluster=w157, "PSC SALES REFERENCES"=w156) -> (w154:T25)
            }
          }
        }
        n123 = local write "Main State"(w11) -> ()
      }
      frame "IDLE" {
        n124 = local write "Main Pages"(T15."IDLE" ("Tab Control")) -> ()
      }
      frame "ADD USER" {
        w175 = Add_User_States."INIT"
        n125 = control-ref of="Add/Edit User Image"() -> (w170:refnum<vi>)
        n126 = while {
          shift-right: [w185] -> _
          shift-left: w175 -> [w188]
          shift-right: [w186] -> _
          shift-left: T36 {"BYU ID #"="", "First Name"="", "Last Name"="", "Phone Number"="", "Email"="", "Department"=0, "Graduation Status"=0, "Anticipated Graduation Year"=0, "Credit Score"="", "Date Added"="", "Graduation Clearance Date"="", "Picture File Name"="", "User Comments"=""} ("USER INFO IN") -> [w187]
          shift-left: w175 -> [w184]
          shift-right: [w182] -> _
          shift-left: T16 refnum ("New Image") -> [w181]
          tunnel: w174 -> [w180]
          tunnel: w170 -> [w179]
          tunnel: [w178] -> w171
          shift-right: [w176] -> w168
          shift-left: w169 -> [w177]
          stop <- w183 stop-if-true
          n127 = case shown="\"END\"" w188 {
            tunnel: w187 -> [w195 w203 w208 w217 w230 w241]
            tunnel: [w194 w203 w208 w217 w229 w239] -> w186
            tunnel: [w197 "ADD USER STATE" w212 w215 w225 Add_User_States."END"] -> w185
            tunnel: w184 -> [_ _ _ _ _ w242]
            tunnel: [FALSE FALSE FALSE FALSE FALSE TRUE] -> w183
            tunnel: [w189 w200 w204 w213 w231 w233] -> w182
            tunnel: w181 -> [_ w200 w206 w219 w231 w234]
            tunnel: w180 -> [w193 _ w207 w220 w228 w238]
            tunnel: w179 -> [w190 _ w205 w214 _ _]
            tunnel: [Main_States."IDLE" Main_States."IDLE" Main_States."IDLE" Main_States."IDLE" Main_States."IDLE" w237] -> w178
            tunnel: w177 -> [w191 w198 w209 w216 w222 w235]
            tunnel: [w191 w198 w209 w216 w222 w236] -> w176
            frame "INIT", Default {
              w197 = Add_User_States."IDLE"
              n128 = call "START ADD USER.vi"("REFERENCES"=w193, "USER INFO IN"=w195) -> ("User Image"=w189:T16, "USER INFO OUT"=w194:T36)  [unwired: 8 in]
              n129 = property class="ImageControl"(reference=w190, "Value"=w189) -> ()  [unwired: 1 in, 2 out]
              n130 = local write "ADD USER STATE"(w197) -> ()
            }
            frame "IDLE" {
            }
            frame "TAKE PHOTO" {
              w212 = Add_User_States."IDLE" ("ADD USER STATE")
              n131 = call "TAKE PHOTO.vi"("Image In"=w206, "REFERENCES"=w207) -> ("Image Out"=w204:T16)  [unwired: 9 in]
              n132 = property class="ImageControl"(reference=w205, "Value"=w204) -> ()  [unwired: 1 in, 2 out]
              n133 = local write "ADD USER STATE"(w212) -> ()
            }
            frame "GET PHOTO" {
              w215 = Add_User_States."IDLE"
              n134 = call "GET ATRIUM PHOTO.vi"("Image In"=w219, "REFERENCES"=w220) -> ("Image Out"=w213:T16)  [unwired: 9 in]
              n135 = property class="ImageControl"(reference=w214, "Value"=w213) -> ()  [unwired: 1 in, 2 out]
              n136 = local write "ADD USER STATE"(w215) -> ()
            }
            frame "ADD USER" {
              w226 = Add_User_States."IDLE"
              n137 = call "UPDATE USER CLUSTER.vi"("REFERENCES"=w228, "USER INFO IN"=w230) -> ("DO NOT PROCEED?"=w224:bool, "USER INFO OUT"=w229:T36)  [unwired: 8 in]
              n138 = local write "ADD USER STATE"(w226) -> ()
              n139 = Select(t=w226, s=w224, f=Add_User_States."END") -> (s? t:f=w225:T14)
            }
            frame "END" {
              n140 = case shown="\"ADD USER\"" w242 {
                tunnel: w241 -> [w247 w252]
                tunnel: [w247 w253] -> w239
                tunnel: w238 -> [_ w254]
                tunnel: [Main_States."IDLE" Main_States."USER ITEMS"] -> w237
                tunnel: [w245 w250] -> w236
                tunnel: w235 -> [w245 _]
                tunnel: w234 -> [w244 w249]
                tunnel: [w244 w248] -> w233
                frame "IDLE", Default {
                }
                frame "ADD USER" {
                  n141 = call "ADD USER TO PGSQL.vi"("Image In"=w249, "REFERENCES"=w254, "USER INFO IN"=w252) -> ("Image Out"=w248:T16, "USER/ITEM DATA TRANSFER"=w250:T1, "USER INFO OUT"=w253:T36)  [unwired: 6 in]
                }
              }
              n142 = call "IMAQ Dispose"() -> ()  [unwired: 6 in, 1 out]
            }
          }
        }
        n143 = local write "Main State"(w171) -> ()
      }
      frame "EDIT USER" {
        w260 = Edit_User_States."INIT"
        n144 = control-ref of="Add/Edit User Image"() -> (w256:refnum<vi>)
        n145 = while {
          shift-right: [w274] -> _
          shift-left: w260 -> [w276]
          shift-left: w260 -> [w270]
          shift-right: [w273] -> _
          shift-left: T36 {"BYU ID #"="", "First Name"="", "Last Name"="", "Phone Number"="", "Email"="", "Department"=0, "Graduation Status"=0, "Anticipated Graduation Year"=0, "Credit Score"="", "Date Added"="", "Graduation Clearance Date"="", "Picture File Name"="", "User Comments"=""} ("USER INFO IN") -> [w275]
          shift-right: [w271] -> _
          shift-left: T16 refnum ("New Image") -> [w272]
          tunnel: w263 -> [w268]
          tunnel: w256 -> [w266]
          tunnel: [Main_States."USER ITEMS"] -> w258
          shift-right: [w264] -> w257
          shift-left: w261 -> [w267]
          stop <- w269 stop-if-true
          n146 = case shown="\"TAKE PHOTO\"" w276 {
            tunnel: w275 -> [_ w287 w295 w303 w313 w322]
            tunnel: [w283 "EDIT USER STATE" w296 w304 w308 Edit_User_States."END"] -> w274
            tunnel: [w281 w287 w295 w303 w312 w321] -> w273
            tunnel: w272 -> [_ w286 w291 w301 w311 w315]
            tunnel: [w277 w286 w289 w297 w311 T16 refnum ("New Image")] -> w271
            tunnel: w270 -> [_ _ _ _ _ w324]
            tunnel: [FALSE FALSE FALSE FALSE FALSE TRUE] -> w269
            tunnel: w268 -> [w280 _ w292 w302 w310 w319]
            tunnel: w267 -> [w279 w284 w293 w299 w305 w318]
            tunnel: w266 -> [w278 _ w290 w298 _ _]
            tunnel: [w279 w284 w293 w299 w305 w317] -> w264
            frame "INIT", Default {
              w283 = Edit_User_States."IDLE"
              n147 = call "START EDIT USER.vi"("USER/ITEM DATA TRANSFER"=w279, "REFERENCES"=w280) -> ("User Image"=w277:T16, "USER INFO OUT"=w281:T36)  [unwired: 8 in]
              n148 = local write "EDIT USER STATE"(w283) -> ()
              n149 = property class="ImageControl"(reference=w278, "Value"=w277) -> ()  [unwired: 1 in, 2 out]
            }
            frame "IDLE" {
            }
            frame "TAKE PHOTO" {
              w296 = Edit_User_States."IDLE"
              n150 = call "TAKE PHOTO.vi"("Image In"=w291, "REFERENCES"=w292) -> ("Image Out"=w289:T16)  [unwired: 9 in]
              n151 = local write "EDIT USER STATE"(w296) -> ()
              n152 = property class="ImageControl"(reference=w290, "Value"=w289) -> ()  [unwired: 1 in, 2 out]
            }
            frame "GET PHOTO" {
              w304 = Edit_User_States."IDLE"
              n153 = call "GET ATRIUM PHOTO.vi"("Image In"=w301, "REFERENCES"=w302) -> ("Image Out"=w297:T16)  [unwired: 9 in]
              n154 = property class="ImageControl"(reference=w298, "Value"=w297) -> ()  [unwired: 1 in, 2 out]
              n155 = local write "EDIT USER STATE"(w304) -> ()
            }
            frame "EDIT USER" {
              w306 = Edit_User_States."IDLE"
              n156 = call "UPDATE USER CLUSTER.vi"("REFERENCES"=w310, "USER INFO IN"=w313) -> ("DO NOT PROCEED?"=w309:bool, "USER INFO OUT"=w312:T36)  [unwired: 8 in]
              n157 = local write "EDIT USER STATE"(w306) -> ()
              n158 = Select(t=w306, s=w309, f=Edit_User_States."END") -> (s? t:f=w308:T13)
            }
            frame "END" {
              n159 = case shown="\"EDIT USER\"" w324 {
                tunnel: w322 -> [w330 w332]
                tunnel: [w329 w332] -> w321
                tunnel: w319 -> [w328 _]
                tunnel: w318 -> [w327 w331]
                tunnel: [w326 w331] -> w317
                tunnel: w315 -> [w325 _]
                frame "EDIT USER" {
                  n160 = call "EDIT USER IN PGSQL.vi"("USER/ITEM DATA TRANSFER IN"=w327, "REFERENCES"=w328, "USER INFO IN"=w330, "Image In"=w325) -> ("USER/ITEM DATA TRANSFER OUT"=w326:T1, "USER INFO OUT"=w329:T36)  [unwired: 6 in]
                }
                frame "IDLE", Default {
                }
              }
            }
          }
        }
        n161 = local write "Main State"(w258) -> ()
      }
      frame "ADD ITEM" {
        w336 = Add_Item_States."INIT"
        n162 = while {
          shift-right: [w344] -> _
          shift-left: T37 {"Identifier"="", "BYU ICN #"="", "Item Description"="", "Comments"="", "Checked Out Date"="", "Due Date"="", "Check Out Location"="", "Reminder Count"="", "Most Recent Reminder Date"="", "BYU ID #"="", "Building/Room"="", "Location in Room"="", "Manual"="", "Manufacturer"="", "Model #"="", "Serial #"="", "Date Acquired"="", "Reminder Notes"=""} ("ITEM DATA IN") -> [w345]
          shift-right: [w342] -> _
          shift-left: w336 -> [w346]
          shift-left: w336 -> [w343]
          tunnel: w338 -> [w340]
          tunnel: [Main_States."IDLE"] -> w335
          stop <- w341 stop-if-true
          n163 = case shown="\"END\"" w346 {
            tunnel: w345 -> [w349 w353 w359 w365]
            tunnel: [w348 w353 w358 w364] -> w344
            tunnel: [w351 "ADD ITEM STATE" w356 Add_Item_States."END"] -> w342
            tunnel: w343 -> [_ _ _ w366]
            tunnel: [FALSE FALSE FALSE TRUE] -> w341
            tunnel: w340 -> [w347 _ w357 _]
            frame "INIT", Default {
              w351 = Add_Item_States."IDLE"
              n164 = call "START ADD ITEM.vi"("REFERENCES"=w347, "ITEM DATA IN"=w349) -> ("ITEM DATA OUT"=w348:T37)  [unwired: 9 in]
              n165 = local write "ADD ITEM STATE"(w351) -> ()
            }
            frame "IDLE" {
            }
            frame "ADD ITEM" {
              n166 = call "UPDATE ITEM CLUSTER.vi"("REFERENCES"=w357, "ITEM DATA IN"=w359) -> ("NO DUPLICATES?"=w355:bool, "ITEM DATA OUT"=w358:T37)  [unwired: 8 in]
              n167 = case shown="True" w355 {
                tunnel: [Add_Item_States."END" w362] -> w356
                frame False {
                }
                frame True {
                  w362 = Add_Item_States."IDLE"
                  n168 = local write "ADD ITEM STATE"(w362) -> ()
                }
              }
              n169 = call "ME # Already Exists"("Enable"=w355) -> ()  [unwired: 9 in, 2 out]
            }
            frame "END" {
              n170 = case shown="\"ADD ITEM\"" w366 {
                tunnel: w365 -> [w369 w370]
                tunnel: [w368 w370] -> w364
                frame "ADD ITEM" {
                  n171 = call "ADD ITEM TO PGSQL.vi"("ITEM DATA IN"=w369) -> ("ITEM DATA OUT"=w368:T37)  [unwired: 10 in]
                }
                frame "IDLE", Default {
                }
              }
            }
          }
        }
        n172 = local write "Main State"(w335) -> ()
      }
      frame "EDIT ITEM" {
        w373 = Edit_Item_States."INIT" ("Enum")
        n173 = while {
          shift-right: [w384] -> _
          shift-left: w373 -> [w385]
          shift-left: w373 -> [w383]
          shift-right: [w382] -> _
          shift-left: T37 {"Identifier"="", "BYU ICN #"="", "Item Description"="", "Comments"="", "Checked Out Date"="", "Due Date"="", "Check Out Location"="", "Reminder Count"="", "Most Recent Reminder Date"="", "BYU ID #"="", "Building/Room"="", "Location in Room"="", "Manual"="", "Manufacturer"="", "Model #"="", "Serial #"="", "Date Acquired"="", "Reminder Notes"=""} ("ITEM DATA IN") -> [w381]
          tunnel: w376 -> [w379]
          tunnel: w374 -> [w378]
          tunnel: [Main_States."IDLE"] -> w372
          stop <- w380 stop-if-true
          n174 = case shown="\"IDLE\"" w385 {
            tunnel: w381 -> [_ w392 w396 w401 w409]
            tunnel: [w390 "EDIT ITEM STATE" w394 w399 Edit_Item_States."END" ("Enum")] -> w384
            tunnel: [w388 w392 w397 w402 w408] -> w382
            tunnel: w383 -> [_ _ _ _ w406]
            tunnel: [FALSE FALSE FALSE FALSE TRUE] -> w380
            tunnel: w379 -> [w387 _ w395 w400 w405]
            tunnel: w378 -> [w386 _ _ _ w404]
            frame "INIT", Default {
              w390 = Edit_Item_States."IDLE" ("Enum")
              n175 = call "START EDIT ITEM.vi"("USER/ITEM DATA TRANSFER IN"=w386, "REFERENCES"=w387) -> ("ITEM DATA OUT"=w388:T37)  [unwired: 9 in]
              n176 = local write "EDIT ITEM STATE"(w390) -> ()
            }
            frame "IDLE" {
            }
            frame "EDIT ITEM" {
              w394 = Edit_Item_States."END" ("Enum")
              n177 = call "UPDATE ITEM CLUSTER.vi"("REFERENCES"=w395, "ITEM DATA IN"=w396) -> ("ITEM DATA OUT"=w397:T37)  [unwired: 8 in, 1 out]
              n178 = local write "EDIT ITEM STATE"(w394) -> ()
            }
            frame "ARCHIVE ITEM" {
              w399 = Edit_Item_States."END" ("Enum")
              n179 = call "UPDATE ITEM CLUSTER.vi"("REFERENCES"=w400, "ITEM DATA IN"=w401) -> ("ITEM DATA OUT"=w402:T37)  [unwired: 8 in, 1 out]
              n180 = local write "EDIT ITEM STATE"(w399) -> ()
            }
            frame "END" {
              n181 = case shown="\"IDLE\", Default" w406 {
                tunnel: w409 -> [w413 w416 w417]
                tunnel: [T37 {"Identifier"="", "BYU ICN #"="", "Item Description"="", "Comments"="", "Checked Out Date"="", "Due Date"="", "Check Out Location"="", "Reminder Count"="", "Most Recent Reminder Date"="", "BYU ID #"="", "Building/Room"="", "Location in Room"="", "Manual"="", "Manufacturer"="", "Model #"="", "Serial #"="", "Date Acquired"="", "Reminder Notes"=""} ("ITEM DATA IN") w415 w417] -> w408
                tunnel: w405 -> [w412 _ _]
                tunnel: w404 -> [_ w414 _]
                frame "ARCHIVE ITEM" {
                  n182 = call "ARCHIVE ITEM.vi"("REFERENCES"=w412, "ITEM DATA IN"=w413) -> ()  [unwired: 10 in]
                }
                frame "EDIT ITEM" {
                  n183 = call "EDIT ITEM IN PGSQL.vi"("USER/ITEM DATA TRANSFER"=w414, "ITEM DATA IN"=w416) -> ("ITEM DATA OUT"=w415:T37)  [unwired: 9 in]
                }
                frame "IDLE", Default {
                }
              }
            }
          }
        }
        n184 = local write "Main State"(w372) -> ()
      }
      frame "RETURN ITEMS" {
        n185 = disable-structure shown="Disabled" {
          disable-tunnel: w421 -> [w424 _]
          disable-tunnel: [FALSE FALSE] -> w420
          disable-tunnel: [w422 w444] -> w418
          frame Disabled {
            n186 = while {
              shift-right: [w429] -> _
              shift-left: Return_Item_States."INIT" -> [w430]
              tunnel: w424 -> [w427]
              tunnel: [Main_States."IDLE"] -> w422
              stop <- w428 stop-if-true
              n187 = case shown="\"RETURN ITEMS\"" w430 {
                tunnel: [w433 "RETURN ITEM STATE" w438 Return_Item_States."SEARCH ITEMS" Return_Item_States."END"] -> w429
                tunnel: [FALSE FALSE FALSE FALSE TRUE] -> w428
                tunnel: w427 -> [w431 _ w436 w439 _]
                frame "INIT", Default {
                  w433 = Return_Item_States."IDLE"
                  n188 = call "START RETURN ITEMS.vi"("REFERENCES"=w431) -> ()  [unwired: 11 in]
                  n189 = local write "RETURN ITEM STATE"(w433) -> ()
                }
                frame "IDLE" {
                }
                frame "SEARCH ITEMS" {
                  w438 = Return_Item_States."IDLE"
                  n190 = call "SEARCH PGSQL FOR ITEMS.vi"("REFERENCES"=w436) -> ()  [unwired: 11 in]
                  n191 = local write "RETURN ITEM STATE"(w438) -> ()
                }
                frame "RETURN ITEMS" {
                  n192 = call "RETURN PGSQL ITEMS.vi"("REFERENCES"=w439) -> ()  [unwired: 11 in]
                }
                frame "END" {
                }
              }
            }
            n193 = local write "Main State"(w422) -> ()
          }
          frame Enabled {
            w444 = Main_States."IDLE"
            n194 = local write "Main State"(w444) -> ()
          }
        }
      }
      frame "SEARCH DATABASE" {
        n195 = while {
          shift-right: [w461] -> _
          shift-left: Search_Database_States."INIT" -> [w463]
          tunnel: w450 -> [w462]
          shift-right: [w459] -> _
          shift-left: string[][] [] -> [w458]
          shift-right: [w457] -> w449
          shift-left: w452 -> [w460]
          shift-right: [w454] -> w446
          shift-left: Main_States."IDLE" -> [w455]
          stop <- w456 stop-if-true
          n196 = case shown="\"UPDATE COLUMNS\"" w463 {
            tunnel: w462 -> [w464 _ w476 w483 w493 w506 w518 w520 w526 _]
            tunnel: [w469 "Search Database State" w481 w487 w488 w501 w514 w522 w530 Search_Database_States."END"] -> w461
            tunnel: w460 -> [w468 w473 w479 w486 _ _ w517 w525 w528 w536]
            tunnel: [w467 w472 w480 w482 w495 w508 w516 w524 w527 w535] -> w459
            tunnel: w458 -> [w467 w472 w480 _ w495 w508 w516 w524 w527 w535]
            tunnel: [w468 w473 w479 w486 w492 w505 w517 w525 w528 w536] -> w457
            tunnel: [FALSE FALSE FALSE FALSE FALSE FALSE FALSE FALSE FALSE TRUE] -> w456
            tunnel: w455 -> [w465 w470 w477 w484 w489 w503 w515 w521 w531 w532]
            tunnel: [w465 w470 w477 w484 w491 w502 w515 w521 w531 w532] -> w454
            frame "INIT", Default {
              w469 = Search_Database_States."UPDATE COLUMNS"
              n197 = call "START SEARCH DATABASE.vi"("REFERENCES"=w464) -> ()  [unwired: 11 in]
              n198 = local write "Search Database State"(w469) -> ()
            }
            frame "IDLE" {
            }
            frame "UPDATE COLUMNS" {
              w481 = Search_Database_States."SEARCH DATABASE"
              n199 = local read "COLUMNS TO VIEW"() -> (w475:bool)
              n200 = local write "Search Database State"(w481) -> ()
              n201 = call "UPDATE LIST VIEW.vi"("COLUMNS TO VIEW"=w475, "REFERENCES"=w476) -> ()  [unwired: 10 in]
            }
            frame "SEARCH DATABASE" {
              w487 = Search_Database_States."IDLE"
              n202 = call "SEARCH DATA.vi"("REFERENCES"=w483) -> ("DATA OUT"=w482:string[][])  [unwired: 10 in]
              n203 = call "SELECT DATA.vi"("DATA IN"=w482, "REFERENCES"=w483) -> ()  [unwired: 10 in]
              n204 = local write "Search Database State"(w487) -> ()
            }
            frame "OPEN USER" {
              n205 = call "OPEN USER OR ITEM.vi"("USER OR ITEM"=enum16{"USER", "ITEM"}."USER", "DATA IN"=w495, "REFERENCES"=w493) -> ("INVALID INPUT"=w490:bool, "USER/ITEM DATA TRANSFER"=w492:T1)  [unwired: 7 in]
              n206 = case shown="False" w490 {
                tunnel: [Main_States."USER ITEMS" w499] -> w491
                tunnel: [Search_Database_States."END" Search_Database_States."IDLE"] -> w488
                tunnel: w489 -> [_ w499]
                frame False {
                }
                frame True {
                }
              }
              n207 = local write "Search Database State"(w488) -> ()
            }
            frame "OPEN ITEM" {
              n208 = call "OPEN USER OR ITEM.vi"("USER OR ITEM"=enum16{"USER", "ITEM"}."ITEM", "DATA IN"=w508, "REFERENCES"=w506) -> ("INVALID INPUT"=w504:bool, "USER/ITEM DATA TRANSFER"=w505:T1)  [unwired: 7 in]
              n209 = case shown="True" w504 {
                tunnel: [Main_States."EDIT ITEM" w512] -> w502
                tunnel: [Search_Database_States."END" Search_Database_States."IDLE"] -> w501
                tunnel: w503 -> [_ w512]
                frame False {
                }
                frame True {
                }
              }
              n210 = local write "Search Database State"(w501) -> ()
            }
            frame "RESTORE USER" {
              w514 = Search_Database_States."IDLE"
              n211 = call "RESTORE USER TO DATABASE.vi"("DATA IN"=w516, "REFERENCES"=w518) -> ()  [unwired: 10 in]
              n212 = local write "Search Database State"(w514) -> ()
            }
            frame "PRINT SALE RECEIPT" {
              w522 = Search_Database_States."IDLE"
              n213 = call "PRINT OLD RECEIPT.vi"("REFERENCES"=w520) -> ()  [unwired: 11 in]
              n214 = local write "Search Database State"(w522) -> ()
            }
            frame "EDIT SALE DESCRIPTION" {
              w530 = Search_Database_States."SEARCH DATABASE"
              n215 = call "EDIT SALE DESCRIPTION.vi"("REFERENCES"=w526) -> ()  [unwired: 11 in]
              n216 = local write "Search Database State"(w530) -> ()
            }
            frame "END" {
            }
          }
        }
        n217 = local write "Main State"(w446) -> ()
      }
      frame "USER ITEMS" {
        n218 = while {
          shift-right: [w550] -> _
          shift-left: User_Item_States."INIT" -> [w554]
          tunnel: w543 -> [w553]
          shift-right: [w552] -> w539
          shift-left: Main_States."IDLE" -> [w551]
          shift-right: [w547] -> w538
          shift-left: w541 -> [w549]
          shift-right: [w545] -> _
          shift-left: TRUE ("Auto Reset") -> [w546]
          stop <- w548 stop-if-true
          n219 = case shown="\"INIT\", Default" w554 {
            tunnel: w553 -> [w561 _ w575 w582 w587 w595 w604 w612 w622 w631 w637 w643 _]
            tunnel: [w560 w572 w578 Main_States."EDIT ITEMS" w591 Main_States."TRANSFER ITEMS" w601 w616 w620 Main_States."CHECK OUT ITEMS" Main_States."EDIT USER" Main_States."IDLE" w649] -> w552
            tunnel: w551 -> [w560 w572 w578 _ w591 _ w600 w616 w619 _ _ _ w649]
            tunnel: [w557 w566 w574 w580 w586 w593 w599 w611 w621 w630 w636 w642 w648] -> w550
            tunnel: w549 -> [w562 w571 w576 _ w588 _ _ w613 _ _ _ w644 w651]
            tunnel: [w562 w571 w576 w581 w588 w594 w603 w613 w624 w633 w639 w644 w651] -> w547
            tunnel: [FALSE FALSE FALSE FALSE FALSE FALSE FALSE FALSE FALSE FALSE FALSE FALSE TRUE] -> w548
            tunnel: w546 -> [w556 w565 _ _ _ _ _ _ _ _ _ _ _]
            tunnel: [w556 FALSE ("Auto Reset") FALSE ("Auto Reset") FALSE ("Auto Reset") FALSE ("Auto Reset") FALSE ("Auto Reset") FALSE ("Auto Reset") FALSE ("Auto Reset") FALSE ("Auto Reset") FALSE ("Auto Reset") FALSE ("Auto Reset") FALSE ("Auto Reset") FALSE ("Auto Reset")] -> w545
            frame "INIT", Default {
              w557 = User_Item_States."IDLE"
              n220 = call "Get User Data.vi"("USER/ITEM DATA TRANSFER"=w562, "REFERENCES"=w561) -> ("USER/ITEM DATA TRANSFER OUT"=w559:T1, "REFERENCES OUT"=w558:T25)  [unwired: 8 in]
              n221 = local write "USER ITEMS STATE"(w557) -> ()
              n222 = call "Get User Items.vi"("USER/ITEM DATA TRANSFER"=w559, "REFERENCES"=w558) -> ()  [unwired: 10 in]
              n223 = property on="SEE USER INFO COMMENTS" class="Bool (strict)"("Value"=FALSE ("SEE USER INFO COMMENTS")) -> ()  [unwired: 2 in, 2 out]
            }
            frame "IDLE" {
              n224 = call "Elapsed Time"("Reset"=w565) -> ("Time has Elapsed"=w567:bool)  [unwired: 11 in, 7 out]
              n225 = Select(t=User_Item_States."END", s=w567, f="USER ITEMS STATE") -> (s? t:f=w566:T8)
            }
            frame "GET USER ITEMS" {
              w574 = User_Item_States."IDLE"
              n226 = call "Get User Items.vi"("USER/ITEM DATA TRANSFER"=w576, "REFERENCES"=w575) -> ()  [unwired: 10 in]
              n227 = local write "USER ITEMS STATE"(w574) -> ()
            }
            frame "EDIT SELECTED ITEMS" {
              w580 = User_Item_States."END"
              n228 = call "Get Selected Items.vi"("REFERENCES"=w582) -> ("USER/ITEM DATA TRANSFER"=w581:T1)  [unwired: 10 in]
              n229 = local write "USER ITEMS STATE"(w580) -> ()
            }
            frame "RETURN SELECTED ITEMS" {
              w586 = User_Item_States."GET USER ITEMS"
              n230 = call "Return Items.vi"("Selection"=enum16{"Selection", "All"}."Selection", "REFERENCES"=w587) -> ()  [unwired: 10 in]
              n231 = local write "USER ITEMS STATE"(w586) -> ()
            }
            frame "TRANSFER SELECTED ITEMS" {
              w593 = User_Item_States."END"
              n232 = call "Get Selected Items.vi"("REFERENCES"=w595) -> ("USER/ITEM DATA TRANSFER"=w594:T1)  [unwired: 10 in]
              n233 = local write "USER ITEMS STATE"(w593) -> ()
            }
            frame "EDIT ALL ITEMS" {
              n234 = call "Get All Items.vi"("REFERENCES"=w604) -> ("No Items?"=w602:bool, "USER/ITEM DATA TRANSFER"=w603:T1)  [unwired: 9 in]
              n235 = case shown="True" w602 {
                tunnel: [Main_States."EDIT ITEMS" w609] -> w601
                tunnel: [User_Item_States."END" User_Item_States."IDLE"] -> w599
                tunnel: w600 -> [_ w609]
                frame False {
                }
                frame True {
                }
              }
              n236 = local write "USER ITEMS STATE"(w599) -> ()
            }
            frame "RETURN ALL ITEMS" {
              w611 = User_Item_States."GET USER ITEMS"
              n237 = local write "USER ITEMS STATE"(w611) -> ()
              n238 = call "Return Items.vi"("Selection"=enum16{"Selection", "All"}."All", "REFERENCES"=w612) -> ()  [unwired: 10 in]
            }
            frame "TRANSFER ALL ITEMS" {
              n239 = call "Get All Items.vi"("REFERENCES"=w622) -> ("No Items?"=w618:bool, "USER/ITEM DATA TRANSFER"=w624:T1)  [unwired: 9 in]
              n240 = case shown="True" w618 {
                tunnel: [Main_States."TRANSFER ITEMS" w628] -> w620
                tunnel: [User_Item_States."END" User_Item_States."IDLE"] -> w621
                tunnel: w619 -> [_ w628]
                frame False {
                }
                frame True {
                }
              }
              n241 = local write "USER ITEMS STATE"(w621) -> ()
            }
            frame "CHECK OUT ITEMS" {
              w630 = User_Item_States."END"
              n242 = call "Get BYU ID.vi"("REFERENCES"=w631) -> ("USER/ITEM DATA TRANSFER"=w633:T1)  [unwired: 10 in]
              n243 = local write "USER ITEMS STATE"(w630) -> ()
            }
            frame "EDIT USER" {
              w636 = User_Item_States."END"
              n244 = call "Get BYU ID.vi"("REFERENCES"=w637) -> ("USER/ITEM DATA TRANSFER"=w639:T1)  [unwired: 10 in]
              n245 = local write "USER ITEMS STATE"(w636) -> ()
            }
            frame "ARCHIVE USER" {
              w642 = User_Item_States."END"
              n246 = call "Archive User.vi"("REFERENCES"=w643) -> ()  [unwired: 11 in]
              n247 = local write "USER ITEMS STATE"(w642) -> ()
            }
            frame "END" {
              w648 = User_Item_States."END"
              n248 = local write "USER ITEMS STATE"(w648) -> ()
            }
          }
        }
        n249 = local write "Main State"(w539) -> ()
      }
      frame "EDIT ITEMS" {
        n250 = while {
          shift-right: [w668] -> _
          shift-left: Edit_Items_States."INIT" -> [w672]
          tunnel: w658 -> [w671]
          shift-right: [w669] -> _
          shift-left: T38[] [] ("DATA OUT") -> [w667]
          shift-right: [w664] -> _
          shift-left: "" -> [w665]
          shift-right: [w663] -> w656
          shift-left: w652 -> [w670]
          shift-right: [w662] -> w654
          shift-left: Main_States."USER ITEMS" -> [w661]
          stop <- w666 stop-if-true
          n251 = case shown="\"EDIT ITEM DESCRIPTION\"" w672 {
            tunnel: w671 -> [w679 _ w695 w700 w706 w715 w726 _ _]
            tunnel: w670 -> [w676 w686 w692 w704 w710 w718 w724 w733 _]
            tunnel: [w678 w687 w694 w699 w707 w713 w727 w731 w738] -> w669
            tunnel: [w674 "EDIT ITEMS STATE" w690 w698 w705 w716 w722 w730 w736] -> w668
            tunnel: w667 -> [_ w687 w696 w701 w708 w714 w728 w731 w738]
            tunnel: [FALSE w681 FALSE FALSE FALSE FALSE FALSE FALSE TRUE] -> w666
            tunnel: [w676 w686 w692 w704 w710 w718 w724 w733 w739] -> w663
            tunnel: w665 -> [_ w685 w693 w703 w711 w719 w723 w732 w737]
            tunnel: [w675 w685 w693 w703 w711 w719 w723 w732 w737] -> w664
            tunnel: [w673 w682 w689 w697 w712 w720 w721 Main_States."USER ITEMS" w735] -> w662
            tunnel: w661 -> [w673 w683 w689 w697 w712 w720 w721 _ w735]
            frame "INIT", Default {
              w674 = Edit_Items_States."IDLE"
              n252 = call "START EDIT ITEMS.vi"("USER/ITEM DATA TRANSFER"=w676, "REFERENCES"=w679) -> ("BYU ID #"=w675:string, "Data Out"=w678:T38[])  [unwired: 8 in]
              n253 = local write "EDIT ITEMS STATE"(w674) -> ()
            }
            frame "IDLE" {
              w680 = Main_States."END" ("y")
              n254 = local read "Main State"() -> (w684:T7)
              n255 = Equal?(x=w684, y=w680) -> (x = y?=w681:bool)
              n256 = Select(t=w680, s=w681, f=w683) -> (s? t:f=w682:T7)
            }
            frame "EDIT DUE DATE" {
              w690 = Edit_Items_States."IDLE"
              n257 = call "EDIT ITEMS DUE DATE.vi"("DATA IN"=w696, "REFERENCES"=w695) -> ("DATA OUT"=w694:T38[])  [unwired: 8 in]
              n258 = local write "EDIT ITEMS STATE"(w690) -> ()
            }
            frame "EDIT LOCATION" {
              w698 = Edit_Items_States."IDLE"
              n259 = call "EDIT ITEMS CHECK OUT LOCATION.vi"("REFERENCES"=w700, "DATA IN"=w701) -> ("DATA OUT"=w699:T38[])  [unwired: 9 in]
              n260 = local write "EDIT ITEMS STATE"(w698) -> ()
            }
            frame "EDIT NOTES" {
              w705 = Edit_Items_States."IDLE"
              n261 = call "EDIT ITEMS REMINDER NOTES.vi"("REFERENCES"=w706, "DATA IN"=w708) -> ("DATA OUT"=w707:T38[])  [unwired: 9 in]
              n262 = local write "EDIT ITEMS STATE"(w705) -> ()
            }
            frame "EDIT ITEM DESCRIPTION" {
              w716 = Edit_Items_States."IDLE"
              n263 = call "EDIT ITEMS ITEM DESCRIPTION.vi"("REFERENCES"=w715, "DATA IN"=w714) -> ("DATA OUT"=w713:T38[])  [unwired: 9 in]
              n264 = local write "EDIT ITEMS STATE"(w716) -> ()
            }
            frame "REMOVE ITEMS" {
              w722 = Edit_Items_States."IDLE"
              n265 = call "REMOVE ITEMS.vi"("REFERENCES"=w726, "DATA IN"=w728) -> ("DATA OUT"=w727:T38[])  [unwired: 9 in]
              n266 = local write "EDIT ITEMS STATE"(w722) -> ()
            }
            frame "EDIT ITEMS" {
              w730 = Edit_Items_States."END"
              n267 = call "EDIT ITEMS IN PGSQL.vi"("DATA IN"=w731) -> ()  [unwired: 11 in]
              n268 = local write "EDIT ITEMS STATE"(w730) -> ()
            }
            frame "END" {
              w736 = Edit_Items_States."END"
              n269 = call "GET USER ID.vi"("BYU ID IN"=w737) -> ("USER/ITEM DATA TRANSFER"=w739:T1)  [unwired: 10 in]
              n270 = local write "EDIT ITEMS STATE"(w736) -> ()
            }
          }
        }
        n271 = local write "Main State"(w654) -> ()
      }
      frame "CHECK OUT ITEMS" {
        n272 = while {
          shift-right: [w754] -> _
          shift-left: Check_Out_Items_States."INIT" -> [w758]
          tunnel: w747 -> [w757]
          shift-right: [w755] -> _
          shift-left: T38[] [] ("DATA OUT") -> [w756]
          tunnel: [w753] -> w745
          tunnel: w743 -> [w751]
          shift-right: [w750] -> w742
          shift-left: Main_States."USER ITEMS" ("Main State") -> [w749]
          stop <- w752 stop-if-true
          n273 = case shown="\"EDIT ITEM DESCRIPTION\"" w758 {
            tunnel: w757 -> [w763 w770 w777 w786 w792 w800 w807 w811 w819 w832]
            tunnel: w756 -> [w764 w771 w774 w784 w789 w796 w805 w813 w822 w833]
            tunnel: [w764 w771 w773 w782 w788 w795 w804 w810 w817 w833] -> w755
            tunnel: [w760 "CHECK OUT ITEMS STATE" w778 w781 w791 w798 w802 w814 w816 Check_Out_Items_States."END"] -> w754
            tunnel: [w763 w770 w777 w786 w792 w800 w807 w811 w818 w832] -> w753
            tunnel: [FALSE w767 FALSE FALSE FALSE FALSE FALSE FALSE FALSE TRUE] -> w752
            tunnel: w751 -> [w761 _ w775 w783 w790 w797 w803 w812 _ _]
            tunnel: [w759 w768 w779 w780 w787 w794 w801 w809 Main_States."USER ITEMS" ("Main State") w830] -> w750
            tunnel: w749 -> [w759 w766 w779 w780 w787 w794 w801 w809 _ w830]
            frame "INIT", Default {
              w760 = Check_Out_Items_States."IDLE"
              n274 = call "START CHECK OUT ITEMS.vi"("REFERENCES"=w761) -> ()  [unwired: 11 in]
              n275 = local write "CHECK OUT ITEMS STATE"(w760) -> ()
            }
            frame "IDLE" {
              w765 = Main_States."END" ("y")
              n276 = local read "Main State"() -> (w769:T7)
              n277 = Equal?(x=w769, y=w765) -> (x = y?=w767:bool)
              n278 = Select(t=w765, s=w767, f=w766) -> (s? t:f=w768:T7)
            }
            frame "UPDATE SEARCH" {
              w778 = Check_Out_Items_States."IDLE"
              n279 = call "UPDATE SEARCH RESULTS.vi"("REFERENCES"=w775, "DATA IN"=w774) -> ("DATA OUT"=w773:T38[])  [unwired: 9 in]
              n280 = local write "CHECK OUT ITEMS STATE"(w778) -> ()
            }
            frame "ADD ITEM" {
              w781 = Check_Out_Items_States."IDLE"
              n281 = call "ADD ITEM TO CHECKOUT.vi"("REFERENCES"=w783, "DATA IN"=w784) -> ("DATA OUT"=w782:T38[])  [unwired: 9 in]
              n282 = local write "CHECK OUT ITEMS STATE"(w781) -> ()
            }
            frame "EDIT DUE DATE" {
              w791 = Check_Out_Items_States."IDLE"
              n283 = call "EDIT DUE DATE.vi"("DATA IN"=w789, "REFERENCES"=w790) -> ("DATA OUT"=w788:T38[])  [unwired: 8 in]
              n284 = local write "CHECK OUT ITEMS STATE"(w791) -> ()
            }
            frame "EDIT LOCATION" {
              w798 = Check_Out_Items_States."IDLE"
              n285 = call "EDIT CHECK OUT LOCATION.vi"("REFERENCES"=w797, "DATA IN"=w796) -> ("DATA OUT"=w795:T38[])  [unwired: 9 in]
              n286 = local write "CHECK OUT ITEMS STATE"(w798) -> ()
            }
            frame "REMOVE ITEMS" {
              w802 = Check_Out_Items_States."IDLE"
              n287 = call "REMOVE ITEMS FROM CHECKOUT.vi"("REFERENCES"=w803, "DATA IN"=w805) -> ("DATA OUT"=w804:T38[])  [unwired: 9 in]
              n288 = local write "CHECK OUT ITEMS STATE"(w802) -> ()
            }
            frame "EDIT ITEM DESCRIPTION" {
              w814 = Check_Out_Items_States."IDLE"
              n289 = call "ALTER ITEM DESCRIPTION.vi"("REFERENCES"=w812, "DATA IN"=w813) -> ("DATA OUT"=w810:T38[])  [unwired: 9 in]
              n290 = local write "CHECK OUT ITEMS STATE"(w814) -> ()
            }
            frame "CHECK OUT ITEMS" {
              n291 = call "VERIFY DATA.vi"("DATA IN"=w822) -> ("DATA BAD?"=w821:bool, "DATA OUT"=w820:T38[])  [unwired: 9 in]
              n292 = case shown="True" w821 {
                tunnel: w820 -> [w825 w828]
                tunnel: w819 -> [w826 w827]
                tunnel: [w826 w827] -> w818
                tunnel: [w825 w828] -> w817
                tunnel: [Check_Out_Items_States."END" Check_Out_Items_States."IDLE"] -> w816
                frame False {
                  n293 = call "CHECK OUT ITEMS IN PGSQL.vi"("USER/ITEM DATA TRANSFER"=w826, "DATA IN"=w825) -> ()  [unwired: 10 in]
                }
                frame True {
                  n294 = call "CHECK DATA"() -> ()  [unwired: 10 in, 2 out]
                }
              }
              n295 = local write "CHECK OUT ITEMS STATE"(w816) -> ()
            }
            frame "END" {
            }
          }
        }
        n296 = local write "Main State"(w742) -> ()
      }
      frame "TRANSFER ITEMS" {
        w838 = Transfer_Items_States."INIT"
        n297 = while {
          shift-right: [w847] -> w841
          shift-left: w843 -> [w853]
          tunnel: w840 -> [w854]
          shift-right: [w855] -> _
          shift-left: w838 -> [w856]
          shift-right: [w852] -> _
          shift-left: T38[] [] ("DATA OUT") -> [w850]
          shift-right: [w848] -> _
          shift-left: "" -> [w849]
          shift-left: w838 -> [w846]
          shift-right: [w845] -> w836
          shift-left: Main_States."USER ITEMS" -> [w844]
          stop <- w851 stop-if-true
          n298 = case shown="\"TRANSFER ITEMS\"" w856 {
            tunnel: [w858 "TRANSFER ITEMS STATE" w874 w881 w888 w897 Transfer_Items_States."END"] -> w855
            tunnel: w854 -> [w863 _ w879 w886 w893 w900 _]
            tunnel: w853 -> [w862 w871 w878 w882 w895 _ w911]
            tunnel: [w860 w870 w876 w883 w892 w902 w905] -> w852
            tunnel: [FALSE w864 FALSE FALSE FALSE FALSE TRUE] -> w851
            tunnel: w850 -> [_ w870 w876 w883 w894 w903 w905]
            tunnel: w849 -> [_ w869 w877 w884 w891 w901 w909]
            tunnel: [w859 w869 w877 w884 w891 w901 "" ("BYU ID")] -> w848
            tunnel: [w862 w871 w878 w882 w890 w899 w910] -> w847
            tunnel: w846 -> [_ _ _ _ _ _ w912]
            tunnel: [w857 w865 w873 w880 w887 Main_States."USER ITEMS" w904] -> w845
            tunnel: w844 -> [w857 w866 w873 w880 w887 _ w904]
            frame "INIT", Default {
              w858 = Transfer_Items_States."IDLE"
              n299 = call "START TRANSFER ITEMS.vi"("USER/ITEM DATA TRANSFER IN"=w862, "REFERENCES"=w863) -> ("DATA OUT"=w860:T38[], "BYU ID #"=w859:string)  [unwired: 8 in]
              n300 = local write "TRANSFER ITEMS STATE"(w858) -> ()
            }
            frame "IDLE" {
              w867 = Main_States."END" ("y")
              n301 = local read "Main State"() -> (w868:T7)
              n302 = Equal?(x=w868, y=w867) -> (x = y?=w864:bool)
              n303 = Select(t=w867, s=w864, f=w866) -> (s? t:f=w865:T7)
            }
            frame "FIND USER" {
              w874 = Transfer_Items_States."IDLE"
              n304 = call "SEARCH USERS.vi"("REFERENCES"=w879) -> ()  [unwired: 11 in]
              n305 = local write "TRANSFER ITEMS STATE"(w874) -> ()
            }
            frame "CONFIRM SELECTION" {
              n306 = call "CONFIRM SELECTION.vi"("REFERENCES"=w886) -> ("STATE OUT"=w881:T4)  [unwired: 10 in]
              n307 = local write "TRANSFER ITEMS STATE"(w881) -> ()
            }
            frame "REMOVE ITEMS" {
              w888 = Transfer_Items_States."IDLE"
              n308 = call "REMOVE FROM ITEM TRANSFER.vi"("USER/ITEM DATA TRANSFER IN"=w895, "REFERENCES"=w893, "DATA IN"=w894) -> ("USER/ITEM DATA TRANSFER OUT"=w890:T1, "DATA OUT"=w892:T38[])  [unwired: 7 in]
              n309 = local write "TRANSFER ITEMS STATE"(w888) -> ()
            }
            frame "TRANSFER ITEMS" {
              w897 = Transfer_Items_States."END"
              n310 = call "TRANSFER ITEMS.vi"("REFERENCES"=w900, "DATA IN"=w903) -> ("USER/ITEM DATA TRANSFER OUT"=w899:T1, "DATA OUT"=w902:T38[])  [unwired: 8 in]
              n311 = local write "TRANSFER ITEMS STATE"(w897) -> ()
            }
            frame "END" {
              n312 = case shown="\"IDLE\", Default" w912 {
                tunnel: w911 -> [_ w918]
                tunnel: [w913 w918] -> w910
                tunnel: w909 -> [w915 _]
                frame "IDLE", Default {
                  n313 = Bundle(cluster=T39 {"DATA TYPE"=enum."BYU ID", "DATA"=""} ("USER/ITEM DATA TRANSFER"), "DATA TYPE"=enum16{"BYU ID", "ME#/IDENTIFIER", "BYU ICN"}."BYU ID", "DATA"=w915) -> (w914:T39)
                  n314 = Build Array(w914) -> (w913:T1)
                }
                frame "TRANSFER ITEMS", "END" {
                }
              }
            }
          }
        }
        n315 = local write "Main State"(w836) -> ()
      }
      frame "PSC SALES" {
        n316 = while {
          shift-right: [w927] -> _
          shift-left: PSC_Sales_States."INIT" -> [w929]
          tunnel: w922 -> [w928]
          tunnel: [Main_States."IDLE"] -> w919
          stop <- w926 stop-if-true
          n317 = case shown="\"RUN CHARGE\"" w929 {
            tunnel: w928 -> [w933 _ w940 w943 w945 w948 w954 w955 w959 _]
            tunnel: [PSC_Sales_States."SEARCH ITEM LIST" "PSC SALES MAIN STATE" w939 w942 PSC_Sales_States."SEARCH ITEM LIST" ("PSC SALES MAIN STATE") w949 w953 w957 PSC_Sales_States."END" ("PSC SALES MAIN STATE") PSC_Sales_States."END" ("PSC SALES MAIN STATE")] -> w927
            tunnel: [FALSE FALSE FALSE FALSE FALSE FALSE FALSE FALSE FALSE TRUE] -> w926
            frame "INIT", Default {
              n318 = call "START SALES.vi"("REFERENCES"=w933) -> ()  [unwired: 11 in]
              n319 = local write "PSC SALES MAIN STATE"(PSC_Sales_States."IDLE") -> ()
            }
            frame "IDLE" {
              n320 = control-ref of="SAVE SALE AND CLOSE"() -> (w935:refnum<vi>)
              n321 = property class="Bool (strict)"(reference=w935, "DisabledEnum"=T40."Enabled" ("Disabled")) -> ()  [unwired: 1 in, 2 out]
            }
            frame "SEARCH ITEM LIST" {
              w939 = PSC_Sales_States."IDLE" ("PSC SALES MAIN STATE")
              n322 = call "SEARCH ITEM LIST.vi"("REFERENCES"=w940) -> ()  [unwired: 11 in]
              n323 = local write "PSC SALES MAIN STATE"(w939) -> ()
            }
            frame "CUSTOM ITEM" {
              w942 = PSC_Sales_States."IDLE" ("PSC SALES MAIN STATE")
              n324 = call "GET CUSTOM ITEM.vi"("REFERENCES"=w943) -> ()  [unwired: 11 in]
              n325 = local write "PSC SALES MAIN STATE"(w942) -> ()
            }
            frame "GET QUANTITY" {
              n326 = call "GET ITEM AMOUNT.vi"("REFERENCES"=w945) -> ()  [unwired: 11 in]
            }
            frame "REMOVE ITEMS" {
              w949 = PSC_Sales_States."IDLE" ("PSC SALES MAIN STATE")
              n327 = call "REMOVE SALE ITEMS.vi"("REFERENCES"=w948) -> ()  [unwired: 11 in]
              n328 = local write "PSC SALES MAIN STATE"(w949) -> ()
            }
            frame "RUN CHARGE" {
              w953 = PSC_Sales_States."IDLE" ("PSC SALES MAIN STATE")
              n329 = call "RUN CHARGE.vi"("REFERENCES"=w954) -> ()  [unwired: 11 in]
              n330 = control-ref of="SAVE SALE AND CLOSE"() -> (w951:refnum<vi>)
              n331 = local write "PSC SALES MAIN STATE"(w953) -> ()
              n332 = property class="Bool (strict)"(reference=w951, "DisabledEnum"=T40."Disabled and Grayed Out" ("Disabled")) -> ()  [unwired: 1 in, 2 out]
            }
            frame "PRINT RECEIPT" {
              w957 = PSC_Sales_States."IDLE" ("PSC SALES MAIN STATE")
              n333 = call "GENERATE SALE RECEIPT.vi"("REFERENCES"=w955) -> ()  [unwired: 11 in]
              n334 = local write "PSC SALES MAIN STATE"(w957) -> ()
            }
            frame "SAVE SALE" {
              n335 = call "SAVE SALE.vi"("REFERENCES"=w959) -> ()  [unwired: 11 in]
            }
            frame "END" {
            }
          }
        }
        n336 = local write "Main Pages"(T15."PSC SALES" ("Tab Control")) -> ()
        n337 = local write "Main State"(w919) -> ()
      }
      frame "ATRIUM" {
        w963 = Main_States."ATRIUM"
        n338 = local write "Main State"(w963) -> ()
      }
      frame "INVENTORY TRACKING" {
        w967 = Main_States."IDLE"
        n339 = local write "Main State"(w967) -> ()
      }
      frame "SETTINGS" {
        n340 = while {
          shift-right: [w983] -> w974
          shift-left: w975 -> [w983]
          shift-right: [w981] -> w973
          shift-left: w976 -> [w982]
          shift-right: [w980] -> _
          shift-left: Settings_States."INIT" -> [w984]
          tunnel: [Main_States."IDLE"] -> w971
          stop <- w978 stop-if-true
          n341 = case shown="\"REMOVE SALE ITEM\"" w984 {
            tunnel: w982 -> [w987 w990 w996 w1004 w1006 w1010]
            tunnel: [w987 w990 w995 w1004 w1006 w1010] -> w981
            tunnel: [w986 "Settings State" w992 w1003 Settings_States."END" ("Settings State") Settings_States."END" ("Settings State")] -> w980
            tunnel: [FALSE FALSE FALSE FALSE FALSE TRUE] -> w978
            frame "INIT", Default {
              w986 = Settings_States."IDLE"
              n342 = call "START EDIT SETTINGS.vi"("REFERENCES"=w987) -> ()  [unwired: 11 in]
              n343 = local write "Settings State"(w986) -> ()
              n344 = local write "Main Pages"(T15."SETTINGS" ("Tab Control")) -> ()
            }
            frame "IDLE" {
            }
            frame "ADD SALE ITEM" {
              w992 = Settings_States."IDLE" ("Settings State")
              n345 = call "Get New Item Info"() -> ("Item Price"=w994:string, "Item Name"=w993:string, "OK"=w997:bool)  [unwired: 16 in, 1 out]
              n346 = case shown="True" w997 {
                tunnel: w996 -> [w999 w1002]
                tunnel: [w999 w1002] -> w995
                tunnel: w994 -> [_ w1001]
                tunnel: w993 -> [_ w1000]
                frame False {
                }
                frame True {
                  n347 = call "ADD SALE ITEM.vi"("Item Name"=w1000, "Item Price"=w1001, "REFERENCES"=w1002) -> ()  [unwired: 9 in]
                }
              }
              n348 = local write "Settings State"(w992) -> ()
            }
            frame "REMOVE SALE ITEM" {
              w1003 = Settings_States."IDLE" ("Settings State")
              n349 = call "REMOVE SALE ITEM.vi"("REFERENCES"=w1004) -> ()  [unwired: 11 in]
              n350 = local write "Settings State"(w1003) -> ()
            }
            frame "UPDATE SETTINGS" {
              n351 = call "UPDATE SETTINGS.vi"("REFERENCES"=w1006) -> ()  [unwired: 11 in]
            }
            frame "END" {
            }
          }
        }
        n352 = local write "Main State"(w971) -> ()
      }
      frame "REMINDER EMAILS" {
        w1012 = Main_States."IDLE"
        n353 = local write "Main State"(w1012) -> ()
        n354 = case shown="\"ENABLE EMAILS\"" "Enable or Disable Emails \n(Make sure only one computer has this enabled)" {
          frame "ENABLE EMAILS" {
            n355 = call "Email Users.vi"() -> ()  [unwired: 12 in]
          }
          frame "DISABLE EMAILS", Default {
          }
        }
      }
      frame "END" {
      }
    }
  }
  n356 = while {
    stop <- w1021 stop-if-true
    n357 = event shown="[89] \"Altered Item Description\": Value Change" {
      selector: _ -> [_ _ _ _ _ _ _ _ _ _ _ _ _ _ _ _ _ _ _ _ _ _ _ _ _ _ _ _ _ _ _ _ _ _ _ _ _ _ _ _ _ _ _ _ _ _ _ _ _ _ _ _ _ _ _ _ _ _ _ _ _ _ _ _ _ _ _ _ _ _ _ _ _ _ _ _ _ _ _ _ _ _ _ _ _ _ _ _ _ _]
      dyn-events: _ -> [_ _ _ _ _ _ _ _ _ _ _ _ _ _ _ _ _ _ _ _ _ _ _ _ _ _ _ _ _ _ _ _ _ _ _ _ _ _ _ _ _ _ _ _ _ _ _ _ _ _ _ _ _ _ _ _ _ _ _ _ _ _ _ _ _ _ _ _ _ _ _ _ _ _ _ _ _ _ _ _ _ _ _ _ _ _ _ _ _ _]
      timeout: 300 -> [_ _ _ _ _ _ _ _ _ _ _ _ _ _ _ _ _ _ _ _ _ _ _ _ _ _ _ _ _ _ _ _ _ _ _ _ _ _ _ _ _ _ _ _ _ _ _ _ _ _ _ _ _ _ _ _ _ _ _ _ _ _ _ _ _ _ _ _ _ _ _ _ _ _ _ _ _ _ _ _ _ _ _ _ _ _ _ _ _ _]
      tunnel: [_ _ _ _ w1120 w1169 _ _ _ _ _ _ _ _ _ _ _ _ _ _ _ _ _ _ _ _ _ _ _ _ _ _ _ _ _ _ _ _ _ _ _ _ _ _ _ _ _ _ _ _ _ _ _ _ _ _ _ _ _ _ _ _ _ _ _ _ _ _ _ _ _ _ _ _ _ _ _ _ _ _ _ _ _ _ _ _ _ _ _ _] -> w1021
      event Timeout {
        n358 = event-data() -> ()  [unwired: 1 in, 1 out]
        n359 = call "CHECK TIME.vi"("EMAILS SENT IN"="EMAILS SENT?") -> ("SEND EMAILS?"=w1023:bool, "EMAILS SENT OUT"=w1024:bool)  [unwired: 9 in]
        n360 = case shown="False" w1023 {
          frame False {
          }
          frame True {
            n361 = local write "Main State"(Main_States."REMINDER EMAILS" ("Main State")) -> ()
          }
        }
        n362 = local write "EMAILS SENT?"(w1024) -> ()
      }
      event "ADD USER": Mouse Up {
        n363 = event-data() -> ()  [unwired: 1 in, 1 out]
        n364 = local read "Main State"() -> (w1028:T7)
        n365 = case shown="\"SETTINGS\"" w1028 {
          tunnel: [Main_States."INIT" ("Main State") w1031 w1032 w1033 w1035 w1037 w1039 w1041 w1043 w1045 w1048 w1050 w1052 w1053 w1054 w1056 Main_States."END" ("Main State")] -> w1029
          tunnel: Main_States."ADD USER" ("Main State") -> [_ w1031 w1032 w1033 w1035 w1037 w1039 w1041 w1043 w1045 w1048 w1050 w1052 w1053 w1054 w1056 _]
          frame "INIT" {
          }
          frame "IDLE", Default {
          }
          frame "ADD USER" {
          }
          frame "EDIT USER" {
            n366 = local write "EDIT USER STATE"(Edit_User_States."END") -> ()
          }
          frame "ADD ITEM" {
            n367 = local write "ADD ITEM STATE"(Add_Item_States."END") -> ()
          }
          frame "EDIT ITEM" {
            n368 = local write "EDIT ITEM STATE"(Edit_Item_States."END" ("Enum")) -> ()
          }
          frame "RETURN ITEMS" {
            n369 = local write "RETURN ITEM STATE"(Return_Item_States."END") -> ()
          }
          frame "SEARCH DATABASE" {
            n370 = local write "Search Database State"(Search_Database_States."END") -> ()
          }
          frame "USER ITEMS" {
            n371 = local write "USER ITEMS STATE"(User_Item_States."END") -> ()
          }
          frame "EDIT ITEMS" {
            n372 = local write "EDIT ITEMS STATE"(Edit_Items_States."END") -> ()
          }
          frame "CHECK OUT ITEMS" {
            n373 = local write "CHECK OUT ITEMS STATE"(Check_Out_Items_States."END") -> ()
          }
          frame "TRANSFER ITEMS" {
            n374 = local write "TRANSFER ITEMS STATE"(Transfer_Items_States."END") -> ()
          }
          frame "PSC SALES" {
            n375 = One Button Dialog(message="Finish or cancel your sale \nto add a user") -> ()  [unwired: 1 in, 1 out]
          }
          frame "ATRIUM" {
          }
          frame "INVENTORY TRACKING" {
          }
          frame "SETTINGS" {
            n376 = One Button Dialog(message="Finish or cancel your settings changes \nto add a user") -> ()  [unwired: 1 in, 1 out]
          }
          frame "END" {
          }
        }
        n377 = local write "Main State"(w1029) -> ()
      }
      event "SEARCH DATABASE": Mouse Up {
        n378 = event-data() -> ()  [unwired: 1 in, 1 out]
        n379 = local read "Main State"() -> (w1059:T7)
        n380 = case shown="\"IDLE\", Default" w1059 {
          tunnel: [Main_States."INIT" ("Main State") w1062 w1064 w1065 w1067 w1069 w1071 w1073 w1074 w1076 w1079 w1081 w1083 w1084 w1085 w1087 Main_States."END" ("Main State")] -> w1060
          tunnel: Main_States."SEARCH DATABASE" ("Main State") -> [_ w1062 w1064 w1065 w1067 w1069 w1071 w1073 w1074 w1076 w1079 w1081 w1083 w1084 w1085 w1087 _]
          frame "INIT" {
          }
          frame "IDLE", Default {
          }
          frame "ADD USER" {
            n381 = local write "ADD USER STATE"(Add_User_States."END" ("ADD USER STATE")) -> ()
          }
          frame "EDIT USER" {
            n382 = local write "EDIT USER STATE"(Edit_User_States."END") -> ()
          }
          frame "ADD ITEM" {
            n383 = local write "ADD ITEM STATE"(Add_Item_States."END") -> ()
          }
          frame "EDIT ITEM" {
            n384 = local write "EDIT ITEM STATE"(Edit_Item_States."END" ("Enum")) -> ()
          }
          frame "RETURN ITEMS" {
            n385 = local write "RETURN ITEM STATE"(Return_Item_States."END") -> ()
          }
          frame "SEARCH DATABASE" {
          }
          frame "USER ITEMS" {
            n386 = local write "USER ITEMS STATE"(User_Item_States."END") -> ()
          }
          frame "EDIT ITEMS" {
            n387 = local write "EDIT ITEMS STATE"(Edit_Items_States."END") -> ()
          }
          frame "CHECK OUT ITEMS" {
            n388 = local write "CHECK OUT ITEMS STATE"(Check_Out_Items_States."END") -> ()
          }
          frame "TRANSFER ITEMS" {
            n389 = local write "TRANSFER ITEMS STATE"(Transfer_Items_States."END") -> ()
          }
          frame "PSC SALES" {
            n390 = One Button Dialog(message="Finish or cancel your sale \nto search the database") -> ()  [unwired: 1 in, 1 out]
          }
          frame "ATRIUM" {
          }
          frame "INVENTORY TRACKING" {
          }
          frame "SETTINGS" {
            n391 = One Button Dialog(message="Finish or cancel your settings changes \nto search the database") -> ()  [unwired: 1 in, 1 out]
          }
          frame "END" {
          }
        }
        n392 = local write "Main State"(w1060) -> ()
      }
      event "PSC SALES": Mouse Up {
        n393 = event-data() -> ()  [unwired: 1 in, 1 out]
        n394 = local read "Main State"() -> (w1090:T7)
        n395 = case shown="\"EDIT ITEMS\"" w1090 {
          tunnel: [Main_States."INIT" ("Main State") w1093 w1095 w1096 w1098 w1100 w1102 w1104 w1106 w1108 w1111 w1113 w1114 w1115 w1116 w1118 Main_States."END" ("Main State")] -> w1091
          tunnel: Main_States."PSC SALES" ("Main State") -> [_ w1093 w1095 w1096 w1098 w1100 w1102 w1104 w1106 w1108 w1111 w1113 w1114 w1115 w1116 w1118 _]
          frame "INIT" {
          }
          frame "IDLE", Default {
          }
          frame "ADD USER" {
            n396 = local write "ADD USER STATE"(Add_User_States."END" ("ADD USER STATE")) -> ()
          }
          frame "EDIT USER" {
            n397 = local write "EDIT USER STATE"(Edit_User_States."END") -> ()
          }
          frame "ADD ITEM" {
            n398 = local write "ADD ITEM STATE"(Add_Item_States."END") -> ()
          }
          frame "EDIT ITEM" {
            n399 = local write "EDIT ITEM STATE"(Edit_Item_States."END" ("Enum")) -> ()
          }
          frame "RETURN ITEMS" {
            n400 = local write "RETURN ITEM STATE"(Return_Item_States."END") -> ()
          }
          frame "SEARCH DATABASE" {
            n401 = local write "Search Database State"(Search_Database_States."END") -> ()
          }
          frame "USER ITEMS" {
            n402 = local write "USER ITEMS STATE"(User_Item_States."END") -> ()
          }
          frame "EDIT ITEMS" {
            n403 = local write "EDIT ITEMS STATE"(Edit_Items_States."END") -> ()
          }
          frame "CHECK OUT ITEMS" {
            n404 = local write "CHECK OUT ITEMS STATE"(Check_Out_Items_States."END") -> ()
          }
          frame "TRANSFER ITEMS" {
            n405 = local write "TRANSFER ITEMS STATE"(Transfer_Items_States."END") -> ()
          }
          frame "PSC SALES" {
          }
          frame "ATRIUM" {
          }
          frame "INVENTORY TRACKING" {
          }
          frame "SETTINGS" {
            n406 = One Button Dialog(message="Finish or cancel your settings changes \nto open sales") -> ()  [unwired: 1 in, 1 out]
          }
          frame "END" {
          }
        }
        n407 = local write "Main State"(w1091) -> ()
      }
      event "CLOSE": Mouse Up {
        n408 = event-data() -> ()  [unwired: 1 in, 1 out]
        n409 = local read "Main State"() -> (w1122:T7)
        n410 = case shown="\"IDLE\", Default" w1122 {
          selector: w1122 -> [_ _ _ _ _ _ _ _ _ _ w1151 w1154 w1157 w1160 w1162 w1164 _]
          tunnel: [Main_States."INIT" ("Main State") w1127 w1130 w1132 w1135 w1138 w1141 w1144 w1147 w1150 w1151 w1154 w1157 w1160 w1162 w1164 Main_States."END" ("Main State")] -> w1123
          tunnel: Main_States."END" ("Main State") -> [_ w1127 w1130 w1132 w1135 w1138 w1141 w1144 w1147 w1150 _ _ _ _ _ _ _]
          tunnel: [FALSE TRUE TRUE TRUE TRUE TRUE TRUE TRUE TRUE TRUE FALSE FALSE FALSE FALSE FALSE FALSE TRUE] -> w1120
          frame "INIT" {
          }
          frame "IDLE", Default {
          }
          frame "ADD USER" {
            n411 = local write "ADD USER STATE"(Add_User_States."END" ("ADD USER STATE")) -> ()
          }
          frame "EDIT USER" {
            n412 = local write "EDIT USER STATE"(Edit_User_States."END") -> ()
          }
          frame "ADD ITEM" {
            n413 = local write "ADD ITEM STATE"(Add_Item_States."END") -> ()
          }
          frame "EDIT ITEM" {
            n414 = local write "EDIT ITEM STATE"(Edit_Item_States."END" ("Enum")) -> ()
          }
          frame "RETURN ITEMS" {
            n415 = local write "RETURN ITEM STATE"(Return_Item_States."END") -> ()
          }
          frame "SEARCH DATABASE" {
            n416 = local write "Search Database State"(Search_Database_States."END") -> ()
          }
          frame "USER ITEMS" {
            n417 = local write "USER ITEMS STATE"(User_Item_States."END") -> ()
          }
          frame "EDIT ITEMS" {
          }
          frame "CHECK OUT ITEMS" {
            n418 = One Button Dialog(message="Finish or cancel before \nyou can close") -> ()  [unwired: 1 in, 1 out]
          }
          frame "TRANSFER ITEMS" {
            n419 = One Button Dialog(message="Finish or cancel before \nyou can close") -> ()  [unwired: 1 in, 1 out]
          }
          frame "PSC SALES" {
            n420 = One Button Dialog(message="Finish or cancel your sale \nto close") -> ()  [unwired: 1 in, 1 out]
          }
          frame "ATRIUM" {
          }
          frame "INVENTORY TRACKING" {
          }
          frame "SETTINGS" {
            n421 = One Button Dialog(message="Finish or cancel your settings changes \nto close") -> ()  [unwired: 1 in, 1 out]
          }
          frame "END" {
          }
        }
        n422 = local write "Main State"(w1123) -> ()
      }
      event Panel Close? {
        n423 = event-data() -> ()  [unwired: 1 in, 1 out]
        n424 = local read "Main State"() -> (w1172:T7)
        n425 = case shown="\"IDLE\", Default" w1172 {
          selector: w1172 -> [_ _ _ _ _ _ _ _ _ _ w1201 w1204 w1207 w1210 w1212 w1214 _]
          tunnel: [Main_States."INIT" ("Main State") w1177 w1180 w1182 w1185 w1188 w1191 w1194 w1197 w1200 w1201 w1204 w1207 w1210 w1212 w1214 Main_States."END" ("Main State")] -> w1173
          tunnel: Main_States."END" ("Main State") -> [_ w1177 w1180 w1182 w1185 w1188 w1191 w1194 w1197 w1200 _ _ _ _ _ _ _]
          tunnel: [FALSE TRUE TRUE TRUE TRUE TRUE TRUE TRUE TRUE TRUE FALSE FALSE FALSE FALSE FALSE FALSE TRUE] -> w1169
          frame "INIT" {
          }
          frame "IDLE", Default {
          }
          frame "ADD USER" {
            n426 = local write "ADD USER STATE"(Add_User_States."END" ("ADD USER STATE")) -> ()
          }
          frame "EDIT USER" {
            n427 = local write "EDIT USER STATE"(Edit_User_States."END") -> ()
          }
          frame "ADD ITEM" {
            n428 = local write "ADD ITEM STATE"(Add_Item_States."END") -> ()
          }
          frame "EDIT ITEM" {
            n429 = local write "EDIT ITEM STATE"(Edit_Item_States."END" ("Enum")) -> ()
          }
          frame "RETURN ITEMS" {
            n430 = local write "RETURN ITEM STATE"(Return_Item_States."END") -> ()
          }
          frame "SEARCH DATABASE" {
            n431 = local write "Search Database State"(Search_Database_States."END") -> ()
          }
          frame "USER ITEMS" {
            n432 = local write "USER ITEMS STATE"(User_Item_States."END") -> ()
          }
          frame "EDIT ITEMS" {
          }
          frame "CHECK OUT ITEMS" {
            n433 = One Button Dialog(message="Finish or cancel before \nyou can close") -> ()  [unwired: 1 in, 1 out]
          }
          frame "TRANSFER ITEMS" {
            n434 = One Button Dialog(message="Finish or cancel before \nyou can close") -> ()  [unwired: 1 in, 1 out]
          }
          frame "PSC SALES" {
            n435 = One Button Dialog(message="Finish or cancel your sale \nto close") -> ()  [unwired: 1 in, 1 out]
          }
          frame "ATRIUM" {
          }
          frame "INVENTORY TRACKING" {
          }
          frame "SETTINGS" {
            n436 = One Button Dialog(message="Finish or cancel your settings changes \nto close") -> ()  [unwired: 1 in, 1 out]
          }
          frame "END" {
          }
        }
        n437 = local write "Main State"(w1173) -> ()
        n438 = Not(x=w1169) -> (.not. x?=w1170:bool)
        n439 = event-data("Discard?"=w1170) -> ()  [unwired: 1 in, 1 out]
      }
      event "ADD ITEM": Mouse Up {
        n440 = event-data() -> ()  [unwired: 1 in, 1 out]
        n441 = local read "Main State"() -> (w1220:T7)
        n442 = case shown="\"SETTINGS\"" w1220 {
          tunnel: [Main_States."INIT" ("Main State") w1223 w1225 w1226 w1228 w1229 w1231 w1233 w1235 w1237 w1240 w1242 w1244 w1245 w1246 w1248 Main_States."END" ("Main State")] -> w1221
          tunnel: Main_States."ADD ITEM" ("Main State") -> [_ w1223 w1225 w1226 w1228 w1229 w1231 w1233 w1235 w1237 w1240 w1242 w1244 w1245 w1246 w1248 _]
          frame "INIT" {
          }
          frame "IDLE", Default {
          }
          frame "ADD USER" {
            n443 = local write "ADD USER STATE"(Add_User_States."END" ("ADD USER STATE")) -> ()
          }
          frame "EDIT USER" {
            n444 = local write "EDIT USER STATE"(Edit_User_States."END") -> ()
          }
          frame "ADD ITEM" {
          }
          frame "EDIT ITEM" {
            n445 = local write "EDIT ITEM STATE"(Edit_Item_States."END" ("Enum")) -> ()
          }
          frame "RETURN ITEMS" {
            n446 = local write "RETURN ITEM STATE"(Return_Item_States."END") -> ()
          }
          frame "SEARCH DATABASE" {
            n447 = local write "Search Database State"(Search_Database_States."END") -> ()
          }
          frame "USER ITEMS" {
            n448 = local write "USER ITEMS STATE"(User_Item_States."END") -> ()
          }
          frame "EDIT ITEMS" {
            n449 = local write "EDIT ITEMS STATE"(Edit_Items_States."END") -> ()
          }
          frame "CHECK OUT ITEMS" {
            n450 = local write "CHECK OUT ITEMS STATE"(Check_Out_Items_States."END") -> ()
          }
          frame "TRANSFER ITEMS" {
            n451 = local write "TRANSFER ITEMS STATE"(Transfer_Items_States."END") -> ()
          }
          frame "PSC SALES" {
            n452 = One Button Dialog(message="Finish or cancel your sale \nto add and item") -> ()  [unwired: 1 in, 1 out]
          }
          frame "ATRIUM" {
          }
          frame "INVENTORY TRACKING" {
          }
          frame "SETTINGS" {
            n453 = One Button Dialog(message="Finish or cancel your settings changes \nto add and item") -> ()  [unwired: 1 in, 1 out]
          }
          frame "END" {
          }
        }
        n454 = local write "Main State"(w1221) -> ()
      }
      event "SAVE AND CLOSE USER": Mouse Up {
        n455 = event-data() -> ()  [unwired: 1 in, 1 out]
        n456 = local read "ADD/EDIT USER LABEL"() -> (w1250:string)
        n457 = case shown="\"ADD USER\"" w1250 {
          frame "EDIT USER" {
            n458 = local write "EDIT USER STATE"(Edit_User_States."EDIT USER" ("EDIT USER STATE")) -> ()
          }
          frame "ADD USER" {
            n459 = local write "ADD USER STATE"(Add_User_States."ADD USER" ("ADD USER STATE")) -> ()
          }
          frame Default {
          }
        }
      }
      event "CANCEL USER": Mouse Up {
        n460 = event-data() -> ()  [unwired: 1 in, 1 out]
        n461 = local read "ADD/EDIT USER LABEL"() -> (w1253:string)
        n462 = case shown="\"ADD USER\"" w1253 {
          frame "EDIT USER" {
            n463 = local write "EDIT USER STATE"(Edit_User_States."END" ("EDIT USER STATE")) -> ()
          }
          frame "ADD USER" {
            n464 = local write "ADD USER STATE"(Add_User_States."END" ("ADD USER STATE")) -> ()
          }
          frame Default {
          }
        }
      }
      event "TAKE PHOTO USER": Mouse Up {
        n465 = event-data() -> ()  [unwired: 1 in, 2 out]
        n466 = local read "ADD/EDIT USER LABEL"() -> (w1256:string)
        n467 = case shown="\"ADD USER\"" w1256 {
          frame "EDIT USER" {
            n468 = local write "EDIT USER STATE"(Edit_User_States."TAKE PHOTO" ("EDIT USER STATE")) -> ()
          }
          frame "ADD USER" {
            n469 = local write "ADD USER STATE"(Add_User_States."TAKE PHOTO" ("ADD USER STATE")) -> ()
          }
          frame Default {
          }
        }
      }
      event "DOWNLOAD USER PHOTO": Mouse Up {
        n470 = event-data() -> ()  [unwired: 1 in, 2 out]
        n471 = local read "ADD/EDIT USER LABEL"() -> (w1259:string)
        n472 = case shown="\"ADD USER\"" w1259 {
          frame "EDIT USER" {
            n473 = local write "EDIT USER STATE"(Edit_User_States."GET PHOTO" ("EDIT USER STATE")) -> ()
          }
          frame "ADD USER" {
            n474 = local write "ADD USER STATE"(Add_User_States."GET PHOTO" ("ADD USER STATE")) -> ()
          }
          frame Default {
          }
        }
      }
      event "SAVE AND CLOSE ITEM": Mouse Up {
        n475 = event-data() -> ()  [unwired: 1 in, 1 out]
        n476 = local read "ADD/EDIT ITEM LABEL"() -> (w1262:string)
        n477 = case shown="\"ADD ITEM\"" w1262 {
          frame "EDIT ITEM" {
            n478 = local write "EDIT ITEM STATE"(Edit_Item_States."EDIT ITEM" ("EDIT ITEM STATE")) -> ()
          }
          frame "ADD ITEM" {
            n479 = local write "ADD ITEM STATE"(Add_Item_States."ADD ITEM" ("ADD ITEM STATE")) -> ()
          }
          frame Default {
          }
        }
      }
      event "ARCHIVE ITEM": Mouse Up {
        n480 = event-data() -> ()  [unwired: 1 in, 1 out]
        n481 = local write "EDIT ITEM STATE"(Edit_Item_States."ARCHIVE ITEM" ("EDIT ITEM STATE")) -> ()
      }
      event "CANCEL ITEM": Mouse Up {
        n482 = event-data() -> ()  [unwired: 1 in, 1 out]
        n483 = local read "ADD/EDIT ITEM LABEL"() -> (w1266:string)
        n484 = case shown="\"ADD ITEM\"" w1266 {
          frame "EDIT ITEM" {
            n485 = local write "EDIT ITEM STATE"(Edit_Item_States."END" ("EDIT ITEM STATE")) -> ()
          }
          frame "ADD ITEM" {
            n486 = local write "ADD ITEM STATE"(Add_Item_States."END" ("ADD ITEM STATE")) -> ()
          }
          frame Default {
          }
        }
      }
      event "RETURN SELECTED ITEMS": Mouse Up {
        n487 = event-data() -> ()  [unwired: 1 in, 1 out]
        n488 = local write "RETURN ITEM STATE"(Return_Item_States."RETURN ITEMS" ("RETURN ITEM STATE")) -> ()
      }
      event "CANCEL RETURN ITEMS": Mouse Up {
        n489 = event-data() -> ()  [unwired: 1 in, 1 out]
        n490 = local write "RETURN ITEM STATE"(Return_Item_States."END" ("RETURN ITEM STATE")) -> ()
      }
      event "Item", "What are you searching for?": Value Change {
        n491 = event-data() -> ()  [unwired: 1 in, 1 out]
        n492 = local write "RETURN ITEM STATE"(Return_Item_States."SEARCH ITEMS" ("RETURN ITEM STATE")) -> ()
      }
      event "OPEN USER": Mouse Up {
        n493 = event-data() -> ()  [unwired: 1 in, 1 out]
        n494 = local write "Search Database State"(Search_Database_States."OPEN USER" ("Search Database State")) -> ()
      }
      event "OPEN ITEM": Mouse Up {
        n495 = event-data() -> ()  [unwired: 1 in, 1 out]
        n496 = local write "Search Database State"(Search_Database_States."OPEN ITEM" ("Search Database State")) -> ()
      }
      event "CLOSE SEARCH": Mouse Up {
        n497 = event-data() -> ()  [unwired: 1 in, 1 out]
        n498 = local write "Search Database State"(Search_Database_States."END" ("Search Database State")) -> ()
      }
      event "EXPORT TO CLIPBOARD": Mouse Up {
        n499 = event-data() -> ()  [unwired: 1 in, 1 out]
        n500 = control-ref of="Search Database Results"() -> (w1275:refnum<vi>)
        n501 = call "EXPORT LISTBOX TO CLIPBOARD.vi"("LISTBOX REFERENCE IN"=w1275) -> ()  [unwired: 11 in]
      }
      event "RESTORE USER": Mouse Up {
        n502 = event-data() -> ()  [unwired: 1 in, 1 out]
        n503 = local write "Search Database State"(Search_Database_States."RESTORE USER") -> ()
      }
      event "COLUMNS TO VIEW": Value Change {
        n504 = event-data() -> ()  [unwired: 1 in, 1 out]
        n505 = local write "Search Database State"(Search_Database_States."UPDATE COLUMNS" ("Search Database State")) -> ()
      }
      event "Where to Search": Value Change {
        n506 = event-data() -> ()  [unwired: 1 in, 1 out]
        n507 = local write "Search Database State"(Search_Database_States."UPDATE COLUMNS" ("Search Database State")) -> ()
      }
      event "What to Search For:": Value Change {
        n508 = event-data() -> ()  [unwired: 1 in, 1 out]
        n509 = local write "Search Database State"(Search_Database_States."SEARCH DATABASE" ("Search Database State")) -> ()
      }
      event "Column to Search In": Value Change {
        n510 = event-data() -> ()  [unwired: 1 in, 1 out]
        n511 = local write "Search Database State"(Search_Database_States."SEARCH DATABASE" ("Search Database State")) -> ()
      }
      event "Column to Sort By": Value Change {
        n512 = event-data() -> ()  [unwired: 1 in, 1 out]
        n513 = local write "Search Database State"(Search_Database_States."SEARCH DATABASE" ("Search Database State")) -> ()
      }
      event "User Column Selector": Value Change {
        n514 = event-data() -> ()  [unwired: 1 in, 1 out]
        n515 = local write "Search Database State"(Search_Database_States."SEARCH DATABASE" ("Search Database State")) -> ()
      }
      event "User Archive Column Selector": Value Change {
        n516 = event-data() -> ()  [unwired: 1 in, 1 out]
        n517 = local write "Search Database State"(Search_Database_States."UPDATE COLUMNS" ("Search Database State")) -> ()
      }
      event "Sales Tracking Column Selector": Value Change {
        n518 = event-data() -> ()  [unwired: 1 in, 1 out]
        n519 = local write "Search Database State"(Search_Database_States."UPDATE COLUMNS" ("Search Database State")) -> ()
      }
      event "Inventory Column Selector": Value Change {
        n520 = event-data() -> ()  [unwired: 1 in, 1 out]
        n521 = local write "Search Database State"(Search_Database_States."UPDATE COLUMNS" ("Search Database State")) -> ()
      }
      event "Inventory Archive Column Selector": Value Change {
        n522 = event-data() -> ()  [unwired: 1 in, 1 out]
        n523 = local write "Search Database State"(Search_Database_States."UPDATE COLUMNS" ("Search Database State")) -> ()
      }
      event "Checked In Archive Selector": Value Change {
        n524 = event-data() -> ()  [unwired: 1 in, 1 out]
        n525 = local write "Search Database State"(Search_Database_States."UPDATE COLUMNS" ("Search Database State")) -> ()
      }
      event "Dates Greater Than", "Dates Less Than", "Date Range": Value Change {
        n526 = event-data() -> ()  [unwired: 1 in, 1 out]
        n527 = local write "Search Database State"(Search_Database_States."SEARCH DATABASE" ("Search Database State")) -> ()
      }
      event "Edit Sale Description": Mouse Up {
        n528 = event-data() -> ()  [unwired: 1 in, 5 out]
        n529 = local write "Search Database State"(Search_Database_States."EDIT SALE DESCRIPTION") -> ()
      }
      event "EDIT USER": Mouse Up {
        n530 = event-data() -> ()  [unwired: 1 in, 1 out]
        n531 = local write "USER ITEMS STATE"(User_Item_States."EDIT USER" ("USER ITEMS STATE")) -> ()
      }
      event "ARCHIVE USER": Mouse Up {
        n532 = event-data() -> ()  [unwired: 1 in, 1 out]
        n533 = local write "USER ITEMS STATE"(User_Item_States."ARCHIVE USER" ("USER ITEMS STATE")) -> ()
      }
      event "LOG OUT USER": Mouse Up {
        n534 = event-data() -> ()  [unwired: 1 in, 1 out]
        n535 = local write "USER ITEMS STATE"(User_Item_States."END" ("USER ITEMS STATE")) -> ()
      }
      event "USER RETURN SELECTED ITEMS": Mouse Up {
        n536 = event-data() -> ()  [unwired: 1 in, 1 out]
        n537 = local read "User's Checked Out Items"() -> (w1297:i32[])
        n538 = Index Array(array=w1297, index=0) -> (element=w1296:i32)
        n539 = Equal?(x=w1296, y=-1 ("index")) -> (x = y?=w1293:bool)
        n540 = case shown="False" w1293 {
          frame False {
            n541 = call "Return Some Warning"() -> ("YES"=w1298:bool)  [unwired: 10 in, 1 out]
            n542 = case shown="True" w1298 {
              frame False {
              }
              frame True {
                n543 = local write "USER ITEMS STATE"(User_Item_States."RETURN SELECTED ITEMS" ("USER ITEMS STATE")) -> ()
              }
            }
          }
          frame True {
          }
        }
      }
      event "CHECK OUT ITEMS": Mouse Up {
        n544 = event-data() -> ()  [unwired: 1 in, 1 out]
        n545 = local write "USER ITEMS STATE"(User_Item_States."CHECK OUT ITEMS" ("USER ITEMS STATE")) -> ()
      }
      event "TRANSFER SELECTED ITEMS": Mouse Up {
        n546 = event-data() -> ()  [unwired: 1 in, 1 out]
        n547 = local read "User's Checked Out Items"() -> (w1305:i32[])
        n548 = Array Size(array=w1305) -> (size(s)=w1304:i32)
        n549 = Index Array(array=w1305, index=0) -> (element=w1307:i32)
        n550 = Equal To 0?(x=w1304) -> (x = 0?=w1303:bool)
        n551 = Equal?(x=w1307, y=-1 ("index")) -> (x = y?=w1302:bool)
        n552 = Or(x=w1303, y=w1302) -> (x .or. y?=w1301:bool)
        n553 = case shown="True" w1301 {
          frame False {
            n554 = local write "USER ITEMS STATE"(User_Item_States."TRANSFER SELECTED ITEMS" ("USER ITEMS STATE")) -> ()
          }
          frame True {
          }
        }
      }
      event "EDIT SELECTED ITEMS": Mouse Up {
        n555 = event-data() -> ()  [unwired: 1 in, 1 out]
        n556 = local read "User's Checked Out Items"() -> (w1314:i32[])
        n557 = Array Size(array=w1314) -> (size(s)=w1313:i32)
        n558 = Index Array(array=w1314, index=0) -> (element=w1317:i32)
        n559 = Equal To 0?(x=w1313) -> (x = 0?=w1312:bool)
        n560 = Equal?(x=w1317, y=-1 ("index")) -> (x = y?=w1311:bool)
        n561 = Or(x=w1312, y=w1311) -> (x .or. y?=w1310:bool)
        n562 = case shown="False" w1310 {
          frame False {
            n563 = local write "USER ITEMS STATE"(User_Item_States."EDIT SELECTED ITEMS" ("USER ITEMS STATE")) -> ()
          }
          frame True {
          }
        }
      }
      event "CANCEL EDIT ITEMS": Mouse Up {
        n564 = event-data() -> ()  [unwired: 1 in, 1 out]
        n565 = local write "EDIT ITEMS STATE"(Edit_Items_States."END" ("EDIT ITEMS STATE")) -> ()
      }
      event "EDIT ITEMS REMOVE SELECTED ITEMS": Mouse Up {
        n566 = event-data() -> ()  [unwired: 1 in, 1 out]
        n567 = local write "EDIT ITEMS STATE"(Edit_Items_States."REMOVE ITEMS" ("EDIT ITEMS STATE")) -> ()
      }
      event "EDIT ITEMS SAVE AND CLOSE": Mouse Up {
        n568 = event-data() -> ()  [unwired: 1 in, 1 out]
        n569 = local write "EDIT ITEMS STATE"(Edit_Items_States."EDIT ITEMS" ("EDIT ITEMS STATE")) -> ()
      }
      event "TODAY EDIT ITEMS": Mouse Up {
        n570 = event-data() -> ()  [unwired: 1 in, 1 out]
        n571 = call "GET CHECK OUT INFO.vi"("Enum"=General_Check_Out_Options."TODAY") -> ("DUE DATE OUT"=w1322:string)  [unwired: 9 in, 1 out]
        n572 = property on="Edit Items Due Date" class="Custom Calendar (strict)"("Val(Sgnl)"=w1322) -> ()  [unwired: 2 in, 2 out]
      }
      event "EDIT ITEMS END OF SEMESTER": Mouse Up {
        n573 = event-data() -> ()  [unwired: 1 in, 1 out]
        n574 = call "GET CHECK OUT INFO.vi"("Enum"=General_Check_Out_Options."END OF SEMESTER") -> ("DUE DATE OUT"=w1324:string)  [unwired: 9 in, 1 out]
        n575 = property on="Edit Items Due Date" class="Custom Calendar (strict)"("Val(Sgnl)"=w1324) -> ()  [unwired: 2 in, 2 out]
      }
      event "EDIT ITEMS STATICS": Mouse Up {
        n576 = event-data() -> ()  [unwired: 1 in, 1 out]
        n577 = call "GET CHECK OUT INFO.vi"("Enum"=General_Check_Out_Options."STATICS") -> ("LOCATION OUT"=w1326:string, "DUE DATE OUT"=w1327:string)  [unwired: 9 in]
        n578 = property on="Edit Items Due Date" class="Custom Calendar (strict)"("Val(Sgnl)"=w1327) -> ()  [unwired: 2 in, 2 out]
        n579 = property on="New Check Out Location" class="Str"("Val(Sgnl)"=w1326) -> ()  [unwired: 2 in, 2 out]
      }
      event "EDIT ITEMS MEASUREMENTS": Mouse Up {
        n580 = event-data() -> ()  [unwired: 1 in, 1 out]
        n581 = call "GET CHECK OUT INFO.vi"("Enum"=General_Check_Out_Options."MEASUREMENTS") -> ("LOCATION OUT"=w1329:string, "DUE DATE OUT"=w1330:string)  [unwired: 9 in]
        n582 = property on="Edit Items Due Date" class="Custom Calendar (strict)"("Val(Sgnl)"=w1330) -> ()  [unwired: 2 in, 2 out]
        n583 = property on="New Check Out Location" class="Str"("Val(Sgnl)"=w1329) -> ()  [unwired: 2 in, 2 out]
      }
      event "EDIT ITEMS MECHATRONICS": Mouse Up {
        n584 = event-data() -> ()  [unwired: 1 in, 1 out]
        n585 = call "GET CHECK OUT INFO.vi"("Enum"=General_Check_Out_Options."MECHATRONICS") -> ("LOCATION OUT"=w1332:string, "DUE DATE OUT"=w1333:string)  [unwired: 9 in]
        n586 = property on="Edit Items Due Date" class="Custom Calendar (strict)"("Val(Sgnl)"=w1333) -> ()  [unwired: 2 in, 2 out]
        n587 = property on="New Check Out Location" class="Str"("Val(Sgnl)"=w1332) -> ()  [unwired: 2 in, 2 out]
      }
      event "CANCEL CHECK OUT ITEMS": Mouse Up {
        n588 = event-data() -> ()  [unwired: 1 in, 1 out]
        n589 = local write "CHECK OUT ITEMS STATE"(Check_Out_Items_States."END" ("CHECK OUT ITEMS STATE")) -> ()
      }
      event "REMOVE SELECTED ITEMS": Mouse Up {
        n590 = event-data() -> ()  [unwired: 1 in, 1 out]
        n591 = local write "CHECK OUT ITEMS STATE"(Check_Out_Items_States."REMOVE ITEMS" ("CHECK OUT ITEMS STATE")) -> ()
      }
      event "FINISH CHECK OUT ITEMS": Mouse Up {
        n592 = event-data() -> ()  [unwired: 1 in, 1 out]
        n593 = local write "CHECK OUT ITEMS STATE"(Check_Out_Items_States."CHECK OUT ITEMS" ("CHECK OUT ITEMS STATE")) -> ()
      }
      event "CHECK OUT END OF SEMESTER": Mouse Up {
        n594 = event-data() -> ()  [unwired: 1 in, 1 out]
        n595 = call "GET CHECK OUT INFO.vi"("Enum"=General_Check_Out_Options."END OF SEMESTER") -> ("DUE DATE OUT"=w1338:string)  [unwired: 9 in, 1 out]
        n596 = property on="Check Out Items Due Date" class="Custom Calendar (strict)"("Val(Sgnl)"=w1338) -> ()  [unwired: 2 in, 2 out]
      }
      event "CHECK OUT MECHATRONICS": Mouse Up {
        n597 = event-data() -> ()  [unwired: 1 in, 1 out]
        n598 = call "GET CHECK OUT INFO.vi"("Enum"=General_Check_Out_Options."MECHATRONICS") -> ("LOCATION OUT"=w1340:string, "DUE DATE OUT"=w1341:string)  [unwired: 9 in]
        n599 = property on="Check Out Items Due Date" class="Custom Calendar (strict)"("Val(Sgnl)"=w1341) -> ()  [unwired: 2 in, 2 out]
        n600 = property on="Check Out Location Selection" class="Str"("Val(Sgnl)"=w1340) -> ()  [unwired: 2 in, 2 out]
      }
      event "CHECK OUT STATICS": Mouse Up {
        n601 = event-data() -> ()  [unwired: 1 in, 1 out]
        n602 = call "GET CHECK OUT INFO.vi"("Enum"=General_Check_Out_Options."STATICS") -> ("LOCATION OUT"=w1343:string, "DUE DATE OUT"=w1344:string)  [unwired: 9 in]
        n603 = property on="Check Out Items Due Date" class="Custom Calendar (strict)"("Val(Sgnl)"=w1344) -> ()  [unwired: 2 in, 2 out]
        n604 = property on="Check Out Location Selection" class="Str"("Val(Sgnl)"=w1343) -> ()  [unwired: 2 in, 2 out]
      }
      event "CHECK OUT MEASUREMENTS": Mouse Up {
        n605 = event-data() -> ()  [unwired: 1 in, 1 out]
        n606 = call "GET CHECK OUT INFO.vi"("Enum"=General_Check_Out_Options."MEASUREMENTS") -> ("LOCATION OUT"=w1346:string, "DUE DATE OUT"=w1347:string)  [unwired: 9 in]
        n607 = property on="Check Out Items Due Date" class="Custom Calendar (strict)"("Val(Sgnl)"=w1347) -> ()  [unwired: 2 in, 2 out]
        n608 = property on="Check Out Location Selection" class="Str"("Val(Sgnl)"=w1346) -> ()  [unwired: 2 in, 2 out]
      }
      event "CHECK OUT TODAY": Mouse Up {
        n609 = event-data() -> ()  [unwired: 1 in, 1 out]
        n610 = call "GET CHECK OUT INFO.vi"("Enum"=General_Check_Out_Options."TODAY") -> ("DUE DATE OUT"=w1349:string)  [unwired: 9 in, 1 out]
        n611 = property on="Check Out Items Due Date" class="Custom Calendar (strict)"("Val(Sgnl)"=w1349) -> ()  [unwired: 2 in, 2 out]
      }
      event "CANCEL TRANSFER ITEMS": Mouse Up {
        n612 = event-data() -> ()  [unwired: 1 in, 1 out]
        n613 = local write "TRANSFER ITEMS STATE"(Transfer_Items_States."END" ("TRANSFER ITEMS STATE")) -> ()
      }
      event "TRANSFER ITEM REMOVE SELECTED ITEMS": Mouse Up {
        n614 = event-data() -> ()  [unwired: 1 in, 1 out]
        n615 = local write "TRANSFER ITEMS STATE"(Transfer_Items_States."REMOVE ITEMS" ("TRANSFER ITEMS STATE")) -> ()
      }
      event "Edit Database Settings": Mouse Up {
        n616 = event-data() -> ()  [unwired: 1 in, 1 out]
        n617 = local write "Main State"(Main_States."SETTINGS" ("Main State")) -> ()
      }
      event "CANCEL EDIT SETTINGS": Mouse Up {
        n618 = event-data() -> ()  [unwired: 1 in, 1 out]
        n619 = local write "Settings State"(Settings_States."END" ("Settings State")) -> ()
      }
      event "Update Settings": Mouse Up {
        n620 = event-data() -> ()  [unwired: 1 in, 1 out]
        n621 = local write "Settings State"(Settings_States."UPDATE SETTINGS" ("Settings State")) -> ()
      }
      event "Matching Individuals": Double Click; "TRANSFER ITEMS": Mouse Up {
        n622 = event-data() -> ()  [unwired: 1 in, 5 out]
        n623 = local write "TRANSFER ITEMS STATE"(Transfer_Items_States."CONFIRM SELECTION" ("TRANSFER ITEMS STATE")) -> ()
      }
      event "Enter Item:": Key Down {
        n624 = event-data() -> ("VKey"=w1360:T42)  [unwired: 1 in]
        n625 = Equal?(x=eventvkey."Enter" ("VKey"), y=w1360) -> (x = y?=w1358:bool)
        n626 = Equal?(x=w1360, y=eventvkey."Return" ("VKey")) -> (x = y?=w1359:bool)
        n627 = Or(x=w1358, y=w1359) -> (x .or. y?=w1357:bool)
        n628 = case shown="False" w1357 {
          frame False {
            n629 = local write "CHECK OUT ITEMS STATE"(Check_Out_Items_States."UPDATE SEARCH" ("CHECK OUT ITEMS STATE")) -> ()
          }
          frame True {
            n630 = local write "CHECK OUT ITEMS STATE"(Check_Out_Items_States."ADD ITEM" ("CHECK OUT ITEMS STATE")) -> ()
          }
        }
      }
      event "Possible Items": Double Click {
        n631 = event-data() -> ()  [unwired: 1 in, 1 out]
        n632 = flat-sequence {
          tunnel: [w1366] -> w1365
          tunnel: w1365 -> [w1375]
          frame #0 {
            n633 = property on="Possible Items" class="MCListbox (strict)"() -> ("ItemNames"=w1371:string[][], "Value"=w1370:i32)  [unwired: 2 in, 2 out]
            n634 = Index Array(array=w1371, index (row)=w1370, index (col)=0 ("disabled index (col)")) -> (element=w1368:string)
            n635 = property on="Enter Item:" class="Str"("Value"=w1368) -> ()  [unwired: 2 in, 2 out]
            n636 = Not Equal?(x=w1368, y="") -> (x != y?=w1366:bool)
          }
          frame #1 {
            n637 = Select(t=Check_Out_Items_States."ADD ITEM" ("CHECK OUT ITEMS STATE"), s=w1375, f=Check_Out_Items_States."IDLE" ("CHECK OUT ITEMS STATE")) -> (s? t:f=w1372:T5)
            n638 = local write "CHECK OUT ITEMS STATE"(w1372) -> ()
          }
        }
      }
      event "Check Out Items Due Date": Value Change {
        n639 = event-data() -> ()  [unwired: 1 in, 1 out]
        n640 = local write "CHECK OUT ITEMS STATE"(Check_Out_Items_States."EDIT DUE DATE" ("CHECK OUT ITEMS STATE")) -> ()
      }
      event "Check Out Location Selection": Value Change {
        n641 = event-data() -> ()  [unwired: 1 in, 1 out]
        n642 = local write "CHECK OUT ITEMS STATE"(Check_Out_Items_States."EDIT LOCATION" ("CHECK OUT ITEMS STATE")) -> ()
      }
      event "Edit Items Due Date": Value Change {
        n643 = event-data() -> ()  [unwired: 1 in, 1 out]
        n644 = local write "EDIT ITEMS STATE"(Edit_Items_States."EDIT DUE DATE" ("EDIT ITEMS STATE")) -> ()
      }
      event "New Check Out Location": Value Change {
        n645 = event-data() -> ()  [unwired: 1 in, 1 out]
        n646 = local write "EDIT ITEMS STATE"(Edit_Items_States."EDIT LOCATION" ("EDIT ITEMS STATE")) -> ()
      }
      event "New Reminder Notes": Value Change {
        n647 = event-data() -> ()  [unwired: 1 in, 5 out]
        n648 = local write "EDIT ITEMS STATE"(Edit_Items_States."EDIT NOTES" ("EDIT ITEMS STATE")) -> ()
      }
      event "New Item Description": Value Change {
        n649 = event-data() -> ()  [unwired: 1 in, 5 out]
        n650 = local write "EDIT ITEMS STATE"(Edit_Items_States."EDIT ITEM DESCRIPTION" ("EDIT ITEMS STATE")) -> ()
      }
      event "Search Parameter", "What to Match": Value Change {
        n651 = event-data() -> ()  [unwired: 1 in, 1 out]
        n652 = local write "TRANSFER ITEMS STATE"(Transfer_Items_States."FIND USER" ("TRANSFER ITEMS STATE")) -> ()
      }
      event "Search Database Results": Double Click {
        n653 = event-data() -> ()  [unwired: 1 in, 1 out]
        n654 = local read "Where to Search"() -> (w1384:u16)
        n655 = case shown="1" w1384 {
          tunnel: [Search_Database_States."OPEN ITEM" Search_Database_States."OPEN USER" Search_Database_States."RESTORE USER" Search_Database_States."IDLE"] -> w1383
          frame 0, 2 {
          }
          frame 1 {
          }
          frame 4 {
          }
          frame Default {
          }
        }
        n656 = local write "Search Database State"(w1383) -> ()
      }
      event "USER EXPORT TO CLIPBOARD": Mouse Up {
        n657 = event-data() -> ()  [unwired: 1 in, 2 out]
        n658 = control-ref of="User's Checked Out Items"() -> (w1389:refnum<vi>)
        n659 = call "EXPORT LISTBOX TO CLIPBOARD.vi"("LISTBOX REFERENCE IN"=w1389) -> ()  [unwired: 11 in]
      }
      event "Scan or Enter Item Name": Value Change {
        n660 = event-data() -> ()  [unwired: 1 in, 2 out]
        n661 = local write "PSC SALES MAIN STATE"(PSC_Sales_States."SEARCH ITEM LIST" ("PSC SALES MAIN STATE")) -> ()
      }
      event "CUSTOM ITEM": Mouse Up {
        n662 = event-data() -> ()  [unwired: 1 in, 2 out]
        n663 = local write "PSC SALES MAIN STATE"(PSC_Sales_States."CUSTOM ITEM" ("PSC SALES MAIN STATE")) -> ()
      }
      event "Item List": Double Click {
        n664 = event-data() -> ()  [unwired: 1 in, 2 out]
        n665 = local write "PSC SALES MAIN STATE"(PSC_Sales_States."GET QUANTITY" ("PSC SALES MAIN STATE")) -> ()
      }
      event "REMOVE SELECTED ITEMS SALES": Mouse Up {
        n666 = event-data() -> ()  [unwired: 1 in, 2 out]
        n667 = local write "PSC SALES MAIN STATE"(PSC_Sales_States."REMOVE ITEMS" ("PSC SALES MAIN STATE")) -> ()
      }
      event "RUN CHARGE": Mouse Up {
        n668 = event-data() -> ()  [unwired: 1 in, 2 out]
        n669 = local write "PSC SALES MAIN STATE"(PSC_Sales_States."RUN CHARGE" ("PSC SALES MAIN STATE")) -> ()
      }
      event "SAVE SALE AND CLOSE": Mouse Up {
        n670 = event-data() -> ()  [unwired: 1 in, 2 out]
        n671 = local write "PSC SALES MAIN STATE"(PSC_Sales_States."SAVE SALE" ("PSC SALES MAIN STATE")) -> ()
      }
      event "CANCEL ITEM SALE": Mouse Up {
        n672 = event-data() -> ()  [unwired: 1 in, 2 out]
        n673 = local write "PSC SALES MAIN STATE"(PSC_Sales_States."END" ("PSC SALES MAIN STATE")) -> ()
      }
      event "ADD NEW SALES ITEM": Mouse Up {
        n674 = event-data() -> ()  [unwired: 1 in, 1 out]
        n675 = local write "Settings State"(Settings_States."ADD SALE ITEM" ("Settings State")) -> ()
      }
      event "REMOVE SALE ITEM": Mouse Up {
        n676 = event-data() -> ()  [unwired: 1 in, 1 out]
        n677 = local write "Settings State"(Settings_States."REMOVE SALE ITEM" ("Settings State")) -> ()
      }
      event "RETURN ITEM": Value Change {
        n678 = event-data() -> ()  [unwired: 1 in, 1 out]
        n679 = control-ref of="USER/ITEM DATA TRANSFER"() -> (w1400:refnum<vi>)
        n680 = control-ref of="RETURN ITEM"() -> (w1401:refnum<vi>)
        n681 = control-ref of="Main State"() -> (w1399:refnum<vi>)
        n682 = call "RETURN ITEM FRONT PANEL.vi"("Main State"=w1399, "USER/ITEM DATA TRANSFER"=w1400, "RETURN ITEM"=w1401) -> ()  [unwired: 9 in]
      }
      event "Items to be Checked Out": Value Change {
        n683 = event-data() -> ()  [unwired: 1 in, 5 out]
        n684 = control-ref of="Items to be Checked Out"() -> (w1403:refnum<vi>)
        n685 = call "CHECK OUT ITEM LOCATION CHECK.vi"("Items Listbox"=w1403) -> ("Change Location"=w1402:bool)  [unwired: 10 in]
        n686 = case shown="True" w1402 {
          frame False {
          }
          frame True {
            n687 = local write "CHECK OUT ITEMS STATE"(Check_Out_Items_States."EDIT LOCATION") -> ()
          }
        }
      }
      event "Print Receipt": Mouse Up {
        n688 = event-data() -> ()  [unwired: 1 in, 5 out]
        n689 = local write "PSC SALES MAIN STATE"(PSC_Sales_States."PRINT RECEIPT" ("PSC SALES MAIN STATE")) -> ()
      }
      event "Search Print Receipt": Mouse Up {
        n690 = event-data() -> ()  [unwired: 1 in, 1 out]
        n691 = local write "Search Database State"(Search_Database_States."PRINT SALE RECEIPT" ("Search Database State")) -> ()
      }
      event "SEE USER INFO COMMENTS": Value Change {
        n692 = event-data() -> ()  [unwired: 1 in, 1 out]
        n693 = property on="User Info Comments" class="Str"("Visible"="SEE USER INFO COMMENTS") -> ()  [unwired: 2 in, 2 out]
      }
      event "Altered Item Description": Value Change {
        n694 = event-data() -> ()  [unwired: 1 in, 1 out]
        n695 = local write "CHECK OUT ITEMS STATE"(Check_Out_Items_States."EDIT ITEM DESCRIPTION") -> ()
      }
    }
  }
